vi "ALONE_3AXIS_V_AMI_DESIM_OLD.vi"(6 "Refresco(s)":dbl=1.0, 8 "error in (no error)":errorcluster) -> (0 "Error Out":errorcluster, 7 "Enable":bool=TRUE)   [LabVIEW 2017]
uses:
  AMI MAGNET/Status AMI.ctl
  AMI MAGNET/magneticField.ctl
  ALONE_3AXIS_AMI.ctl
  AMI MAGNET/commsControl.ctl
  AMI MAGNET/AMI 430_Hardware_Module.ctl
  cRIO_ZNB_AMI_GLOBALES.vi
panel:
  out "Ciclo 2":i32
  out "TIEMPO Y":dbl
  out "TIEMPO X":dbl
  out "TIEMPO Z":dbl
  out "cTarget_X":dbl min=-0.5 max=0.5 step=0.001 format="%.3f"
  out "cRate_X":dbl=0.1 min=0.0 max=0.1 step=0.001 format="%.3f"
  out "cTarget_Y":dbl min=-0.5 max=0.5 step=0.001 format="%.3f"
  out "cRate_Y":dbl=0.1 min=0.0 max=0.1 step=0.001 format="%.3f"
  out "ConfigZ":T1={"connection ID"=refnum, "IP"="192.168.0.106", "Active Comm Interface"=0, "Serial Port"="", "Programmer Type"=0, "connection ID"=refnum, "output cluster"={"GPIB address"=22, "GPIB bus"=1}} {"Programmer Type" items=["Model 430", "Model 420"]; "Active Comm Interface" items=["TCP/IP (Model 430 Only)", "RS232", "IEEE488"]}
  out "ConfigY":T1={"connection ID"=refnum, "IP"="192.168.0.107", "Active Comm Interface"=0, "Serial Port"="", "Programmer Type"=0, "connection ID"=refnum, "output cluster"={"GPIB address"=22, "GPIB bus"=1}} {"Programmer Type" items=["Model 430", "Model 420"]; "Active Comm Interface" items=["TCP/IP (Model 430 Only)", "RS232", "IEEE488"]}
  out "ConfigX":T1={"connection ID"=refnum, "IP"="192.168.0.108", "Active Comm Interface"=0, "Serial Port"="", "Programmer Type"=0, "connection ID"=refnum, "output cluster"={"GPIB address"=22, "GPIB bus"=1}} {"Programmer Type" items=["Model 430", "Model 420"]; "Active Comm Interface" items=["TCP/IP (Model 430 Only)", "RS232", "IEEE488"]}
  in  "DEMAG X":bool
  in  "x":dbl=0.1 min=-0.5 max=0.5 step=0.001 format="%.3f"
  in  "y":dbl=0.2 min=-0.5 max=0.5 step=0.001 format="%.3f"
  in  "GO XYZ":bool
  in  "DEMAG Y":bool
  in  "DEMAG Z":bool
  out "Estado":string
  out "Command":T2
  in  "Mode X":u16(ring) items=["RAMP", "PAUSE", "MANUAL UP", "MANUAL DOWN", "ZERO"]
  in  "Mode Y":u16(ring) items=["RAMP", "PAUSE", "MANUAL UP", "MANUAL DOWN", "ZERO"]
  in  "Mode Z":u16(ring) items=["RAMP", "PAUSE", "MANUAL UP", "MANUAL DOWN", "ZERO"]
  in  "GO Z":bool
  in  "SET X":bool
  out "X ramping":bool caption="Stable"
  out "X state":T3=1 items=["Unknown", "RAMPING to target field/current", "HOLDING at the target field/current", "PAUSED", "Ramping in MANUAL UP mode", "Ramping in MANUAL DOWN mode", "ZEROING CURRENT (in progress)", "Quench detected", "At ZERO current", "Heating persistent switch", "Cooling persistent switch", "External Rampdown active"]
  in  "Target X":dbl caption="Target(T)" min=-0.5 max=0.5 step=0.001 format="%.3f"
  in  "Rate X":dbl=0.1 caption="Rate(T/min)" min=0.0 max=0.1 step=0.001 format="%.3f"
  out "X field":dbl caption="X field (T)" format="%.3f"
  in  "SET Y":bool
  out "Y ramping":bool caption="Stable"
  out "Y state":T3=1 items=["Unknown", "RAMPING to target field/current", "HOLDING at the target field/current", "PAUSED", "Ramping in MANUAL UP mode", "Ramping in MANUAL DOWN mode", "ZEROING CURRENT (in progress)", "Quench detected", "At ZERO current", "Heating persistent switch", "Cooling persistent switch", "External Rampdown active"]
  in  "Target Y":dbl caption="Target(T)" min=-0.5 max=0.5 step=0.001 format="%.3f"
  in  "Rate Y":dbl=0.1 caption="Rate(T/min)" min=0.0 max=0.1 step=0.001 format="%.3f"
  out "Y field":dbl caption="Y field (T)" format="%.3f"
  in  "GO X":bool
  in  "GO Y":bool
  in  "Settings Z":T4={"magneticFieldUnits"=1, "rampRateUnits"=1, "rampRate"=0.0, "targetField"=0.0, "rampingMode"=1} {"rampingMode" items=["RAMP", "PAUSE", "MANUAL UP", "MANUAL DOWN", "ZERO"]; "targetField" format="%.3f"; "rampRate" format="%.3f"; "rampRateUnits" items=["Per SECOND", "Per MINUTE"]; "magneticFieldUnits" items=["KGauss", "Tesla"]}
  in  "Settings Y":T4={"magneticFieldUnits"=1, "rampRateUnits"=1, "rampRate"=0.0, "targetField"=0.0, "rampingMode"=1} {"rampingMode" items=["RAMP", "PAUSE", "MANUAL UP", "MANUAL DOWN", "ZERO"]; "targetField" format="%.3f"; "rampRate" format="%.3f"; "rampRateUnits" items=["Per SECOND", "Per MINUTE"]; "magneticFieldUnits" items=["KGauss", "Tesla"]}
  in  "Settings X":T4={"magneticFieldUnits"=1, "rampRateUnits"=1, "rampRate"=0.0, "targetField"=0.0, "rampingMode"=1} {"rampingMode" items=["RAMP", "PAUSE", "MANUAL UP", "MANUAL DOWN", "ZERO"]; "targetField" format="%.3f"; "rampRate" format="%.3f"; "rampRateUnits" items=["Per SECOND", "Per MINUTE"]; "magneticFieldUnits" items=["KGauss", "Tesla"]}
  out "Waveform Chart":T5(graph)
  in  "SET Z":bool
  out "Z ramping":bool caption="Stable"
  out "Z state":T3=1 items=["Unknown", "RAMPING to target field/current", "HOLDING at the target field/current", "PAUSED", "Ramping in MANUAL UP mode", "Ramping in MANUAL DOWN mode", "ZEROING CURRENT (in progress)", "Quench detected", "At ZERO current", "Heating persistent switch", "Cooling persistent switch", "External Rampdown active"]
  out "Ciclo":i32
  in  "Target Z":dbl caption="Target(T)" min=-2.0 max=2.0 step=0.001 format="%.3f"
  in  "Rate Z":dbl=0.1 caption="Rate(T/min)" min=0.0 max=0.1 step=0.001 format="%.3f"
  out "Z field":dbl caption="Z field (T)" format="%.3f"
  out "Error":bool
  out "Date":string
  out "Time":string
  in  "Refresh":bool
  in  "stop":bool
  # "X axis"
  # "Z axis"
  # "STATUS"
  # "Y axis"
  # "STATUS"
  # "STATUS"
  # "SETTINGS"
  # "SETTINGS"
  # "SETTINGS"
  # "-----------X field = x . Z field------------------------------Y field = y . Z field---------------------------- Enlazar con eje Z -------------"
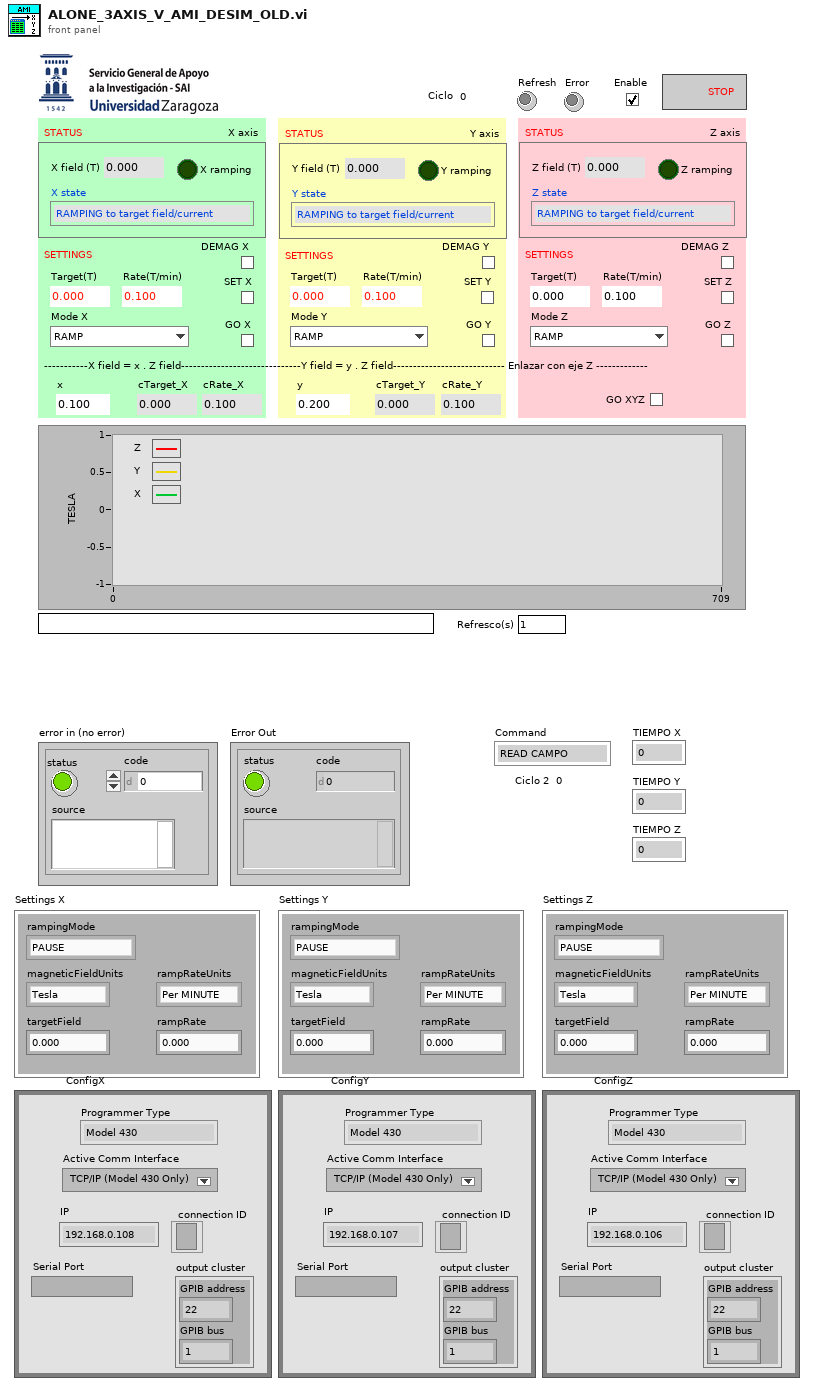
[diagram p1: front panel]
types:
  T1 = typedef "commsControl.ctl" = cluster{"connection ID":refnum<k5>, "IP":string, "Active Comm Interface":u16, "Serial Port":refnum<visa-resource-name>, "Programmer Type":u16, "connection ID":refnum<k5>, "output cluster":cluster{"GPIB address":i16, "GPIB bus":i16}}
  T2 = typedef "ALONE_3AXIS_AMI.ctl" = enum16{"READ CAMPO", "SET X", "SET Y", "SET Z", "RAMP X", "RAMP Y", "RAMP Z", "RAMP XYZ", "DESIMANAR X", "DESIMANAR Y", "DESIMANAR Z", "DESIMANAR X_RUN", "DESIMANAR Y_RUN", "DESIMANAR Z_RUN"}
  T3 = typedef "Status AMI.ctl" = u16
  T4 = typedef "magneticField.ctl" = cluster{"magneticFieldUnits":u16, "rampRateUnits":u16, "rampRate":dbl, "targetField":dbl, "rampingMode":u16}
  T5 = cluster{"magneticField":dbl, "magneticField":dbl, "magneticField":dbl}
  T6 = typedef "AMI 430_Hardware_Module.ctl" = enum16{"INICIALIZAR", "SET UNIDADES CAMPO", "SET UNIDADES RAMPA", "SET CAMPO", "SET  RAMPA", "SET RAMPING MODE", "READ CAMPO", "STATUS", "SHUTDOWN"}
  T7 = cluster{"Z field":dbl, "Y field":dbl, "magneticField":dbl}
  T8 = cluster{"Z field":dbl, "magneticField":dbl, "X field":dbl}
  T9 = cluster{"magneticField":dbl, "Y field":dbl, "X field":dbl}
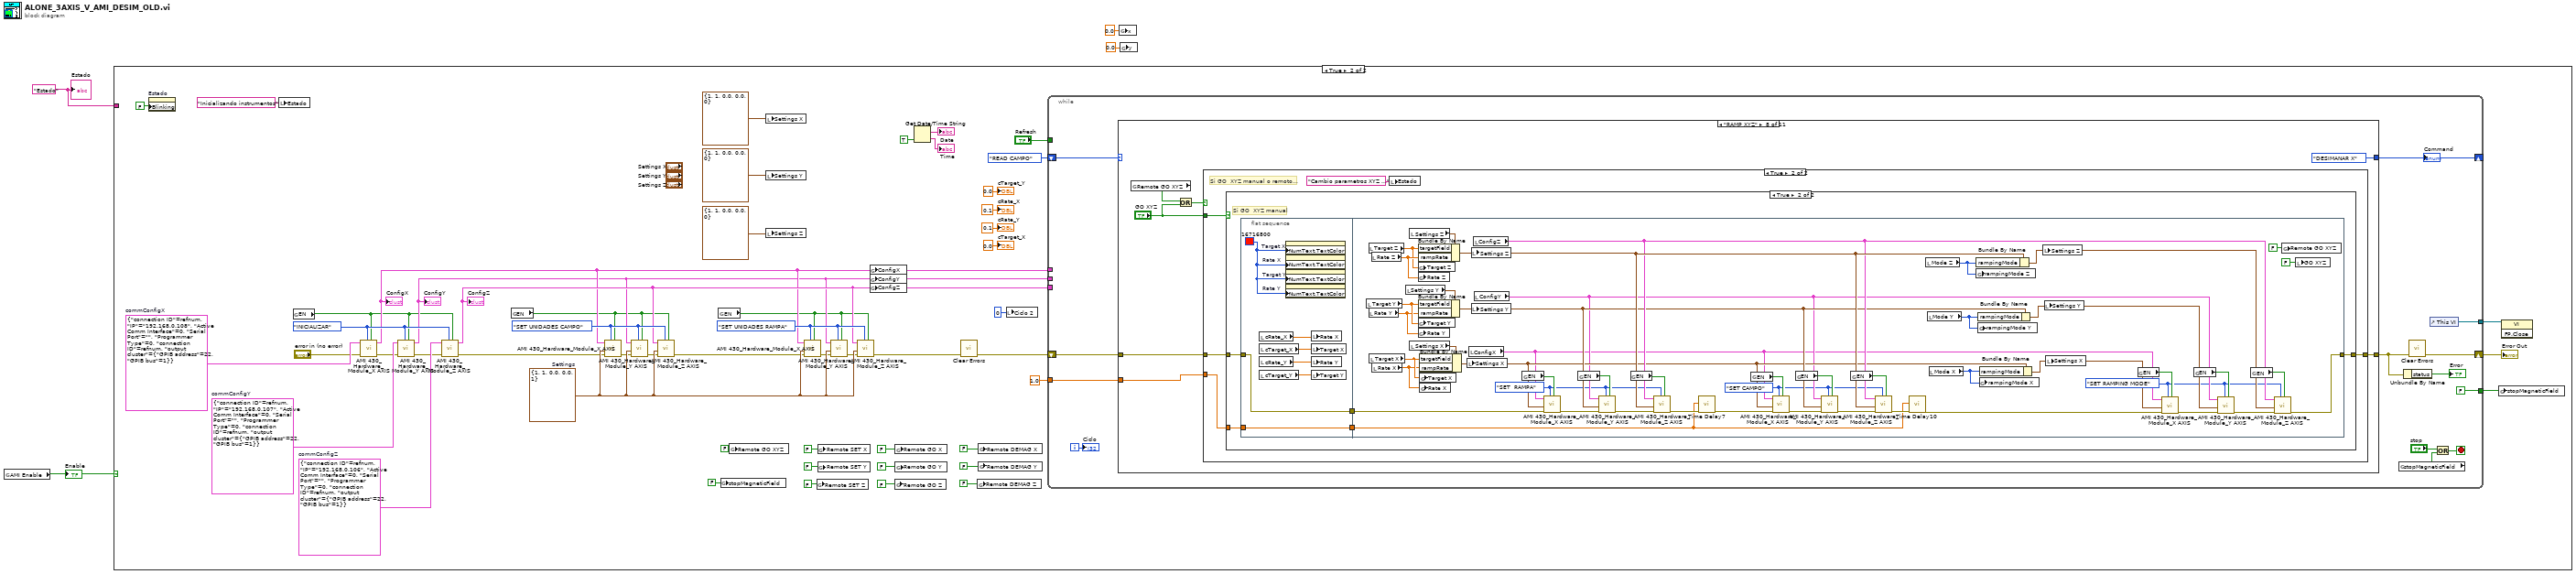
[diagram p0: block diagram]
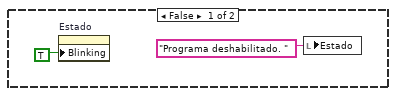
[diagram p2: hidden frame]
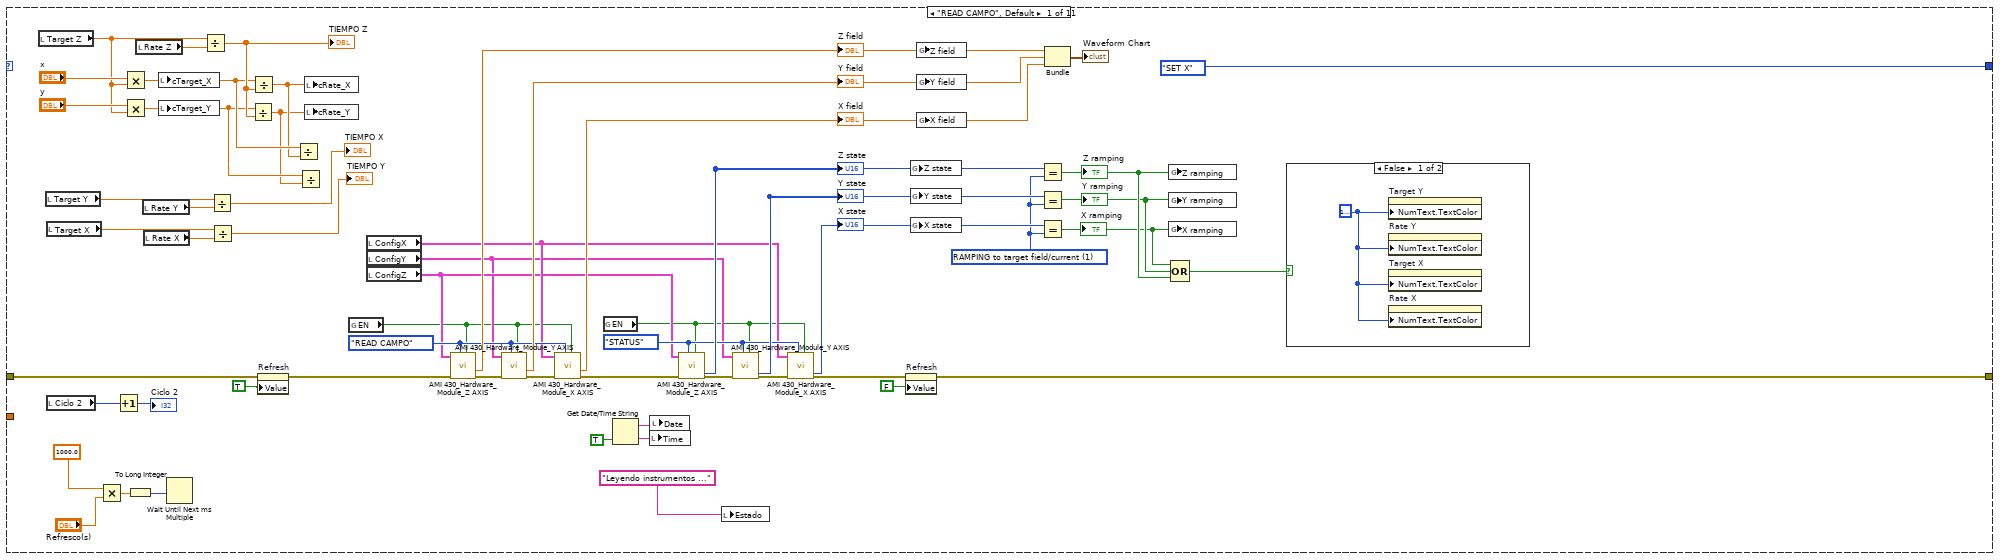
[diagram p3: hidden frame]
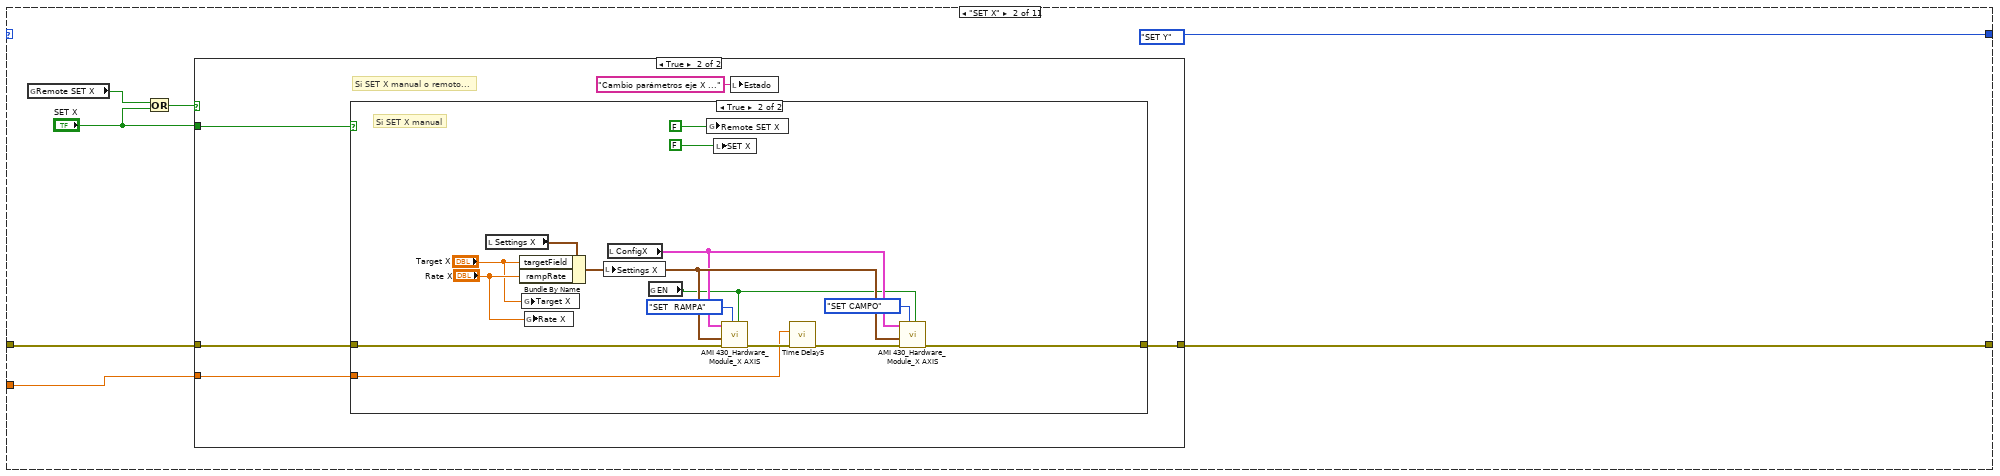
[diagram p5: hidden frame]
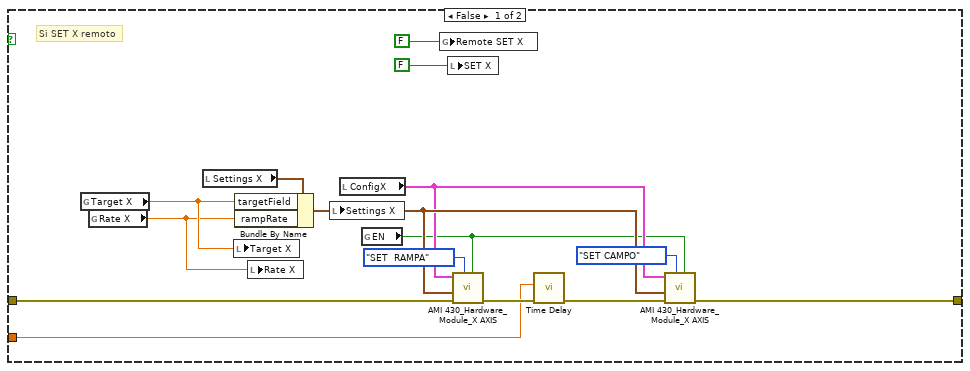
[diagram p7: hidden frame]
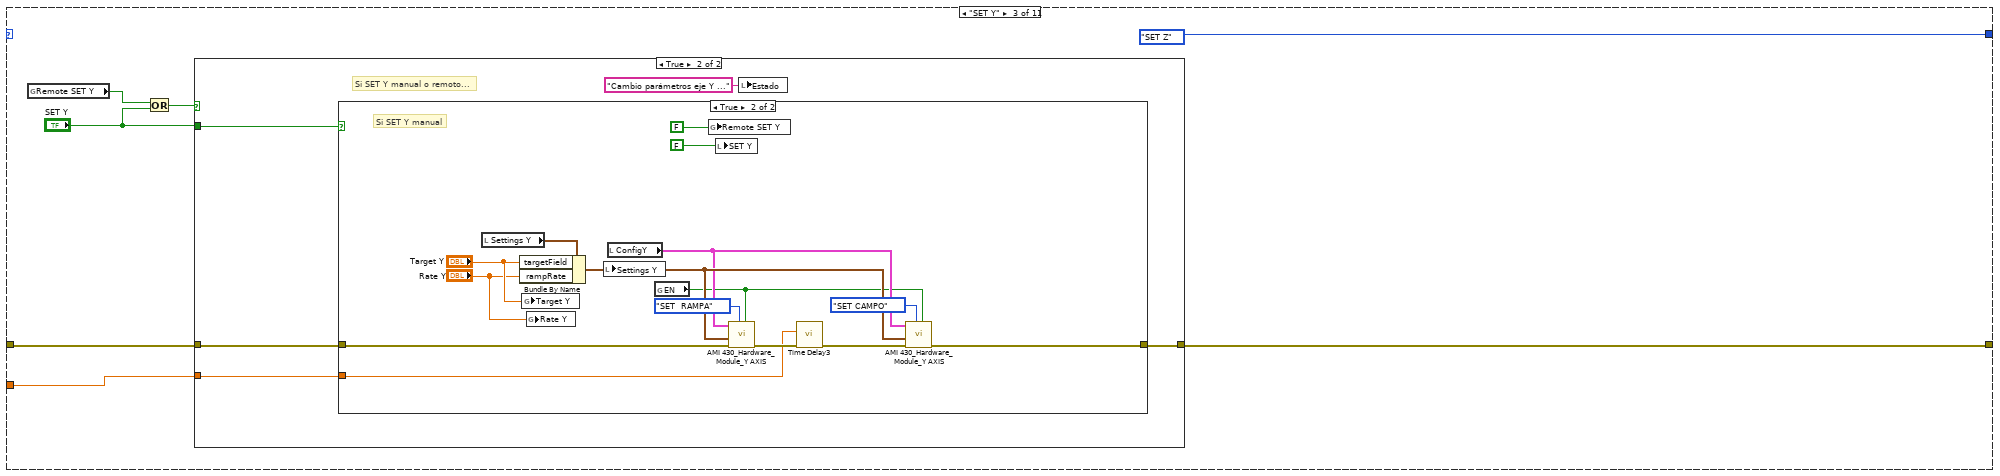
[diagram p8: hidden frame]
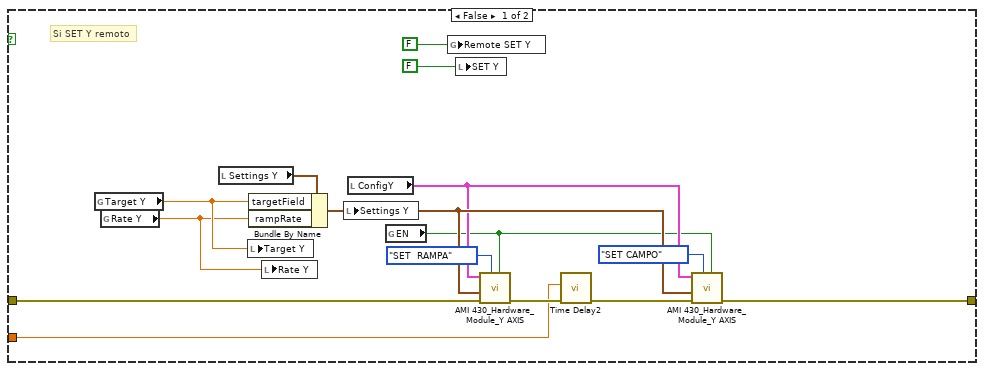
[diagram p10: hidden frame]
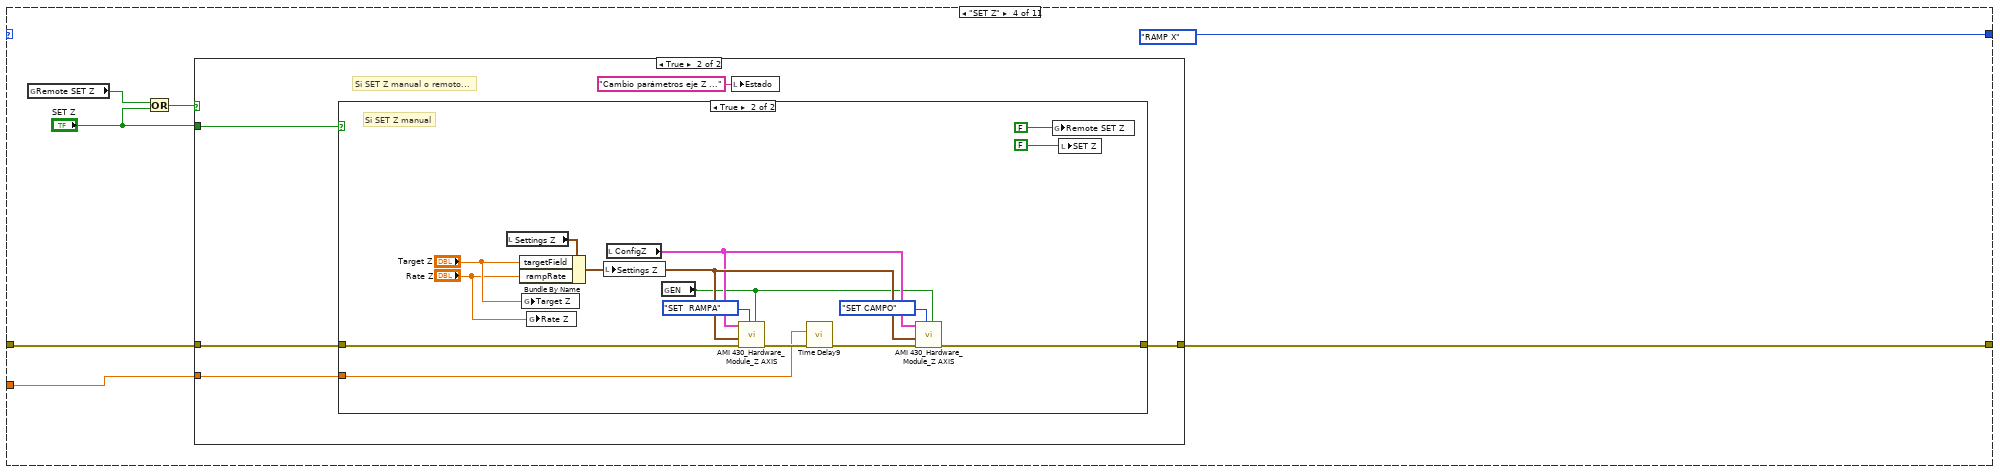
[diagram p11: hidden frame]
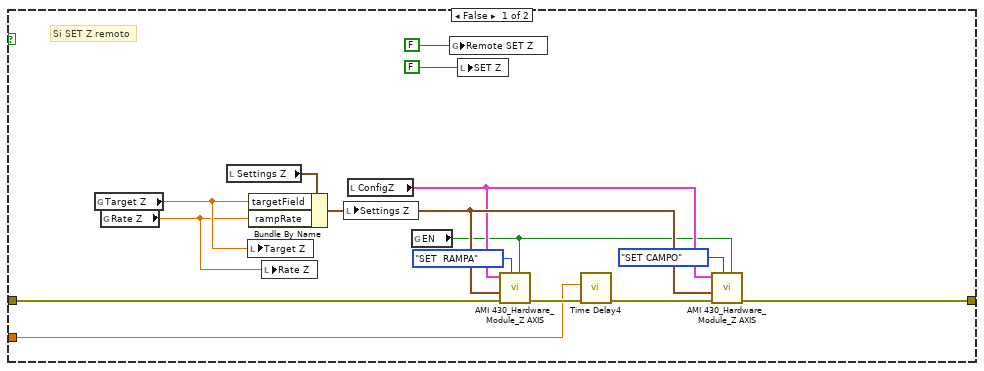
[diagram p13: hidden frame]
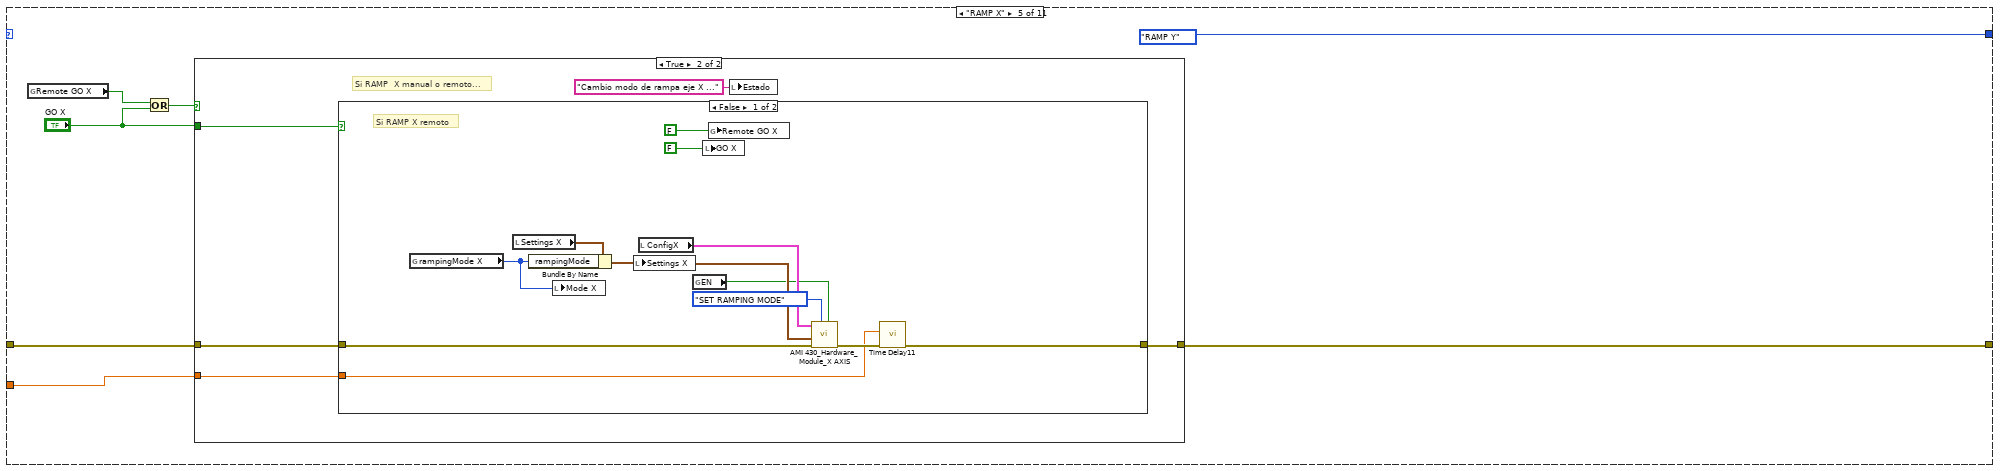
[diagram p14: hidden frame]
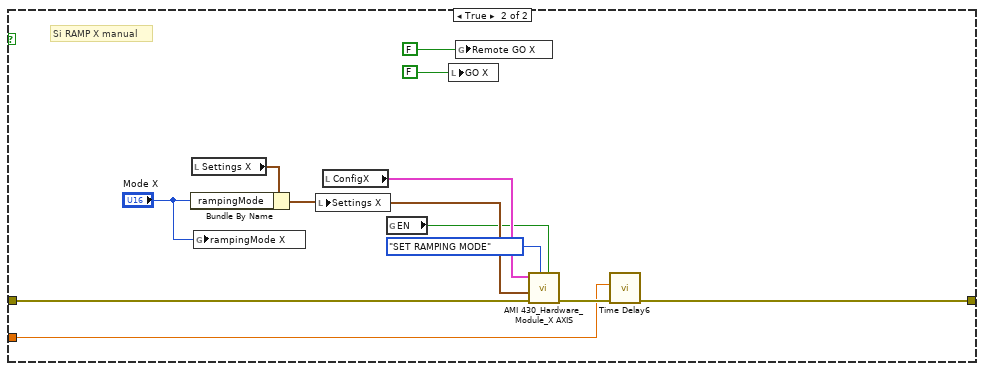
[diagram p16: hidden frame]
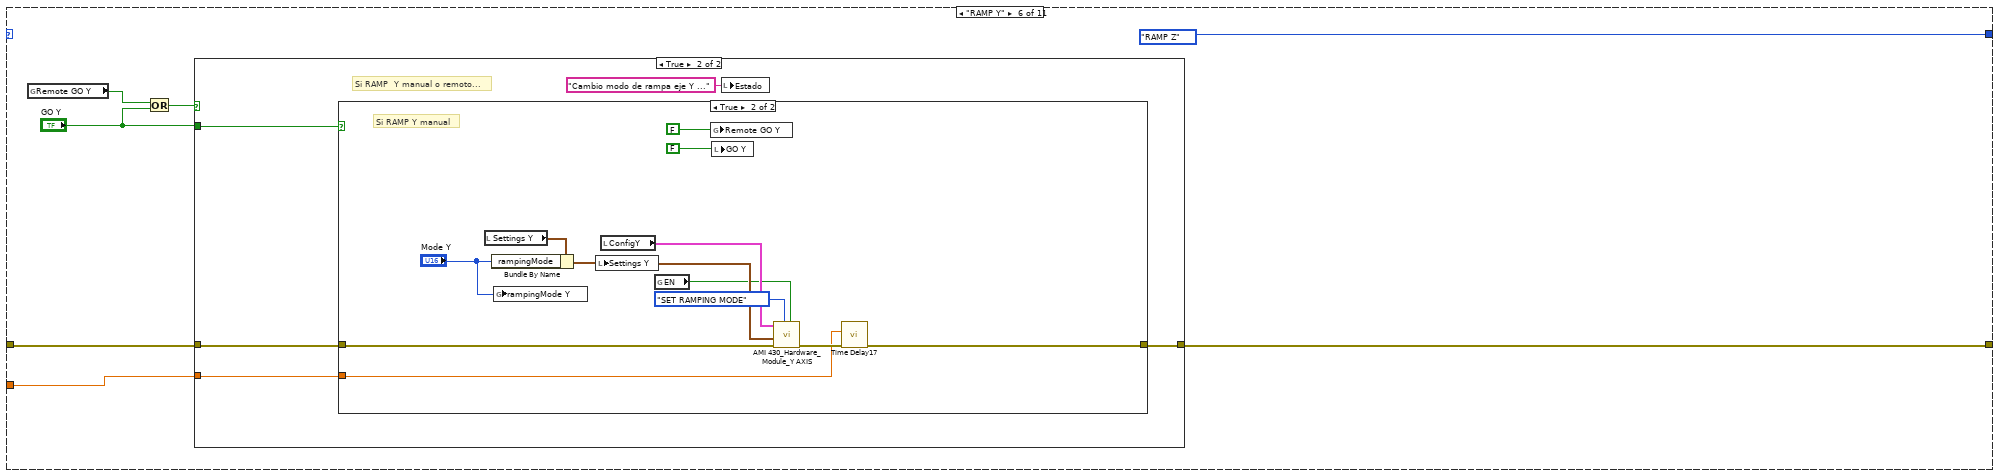
[diagram p17: hidden frame]
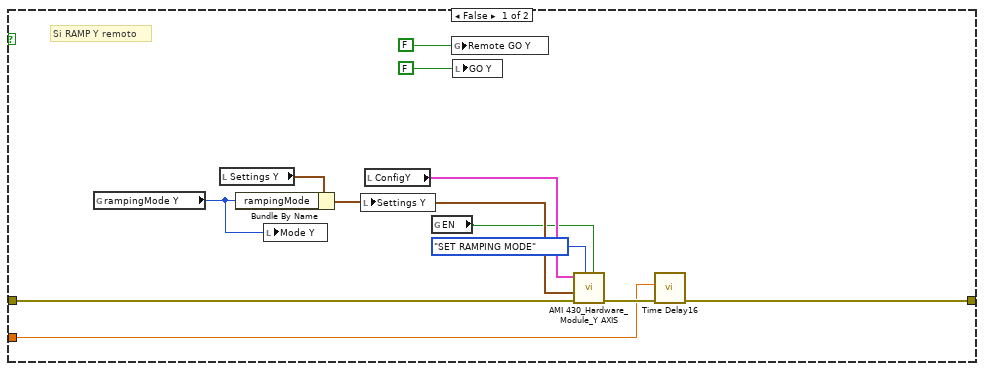
[diagram p19: hidden frame]
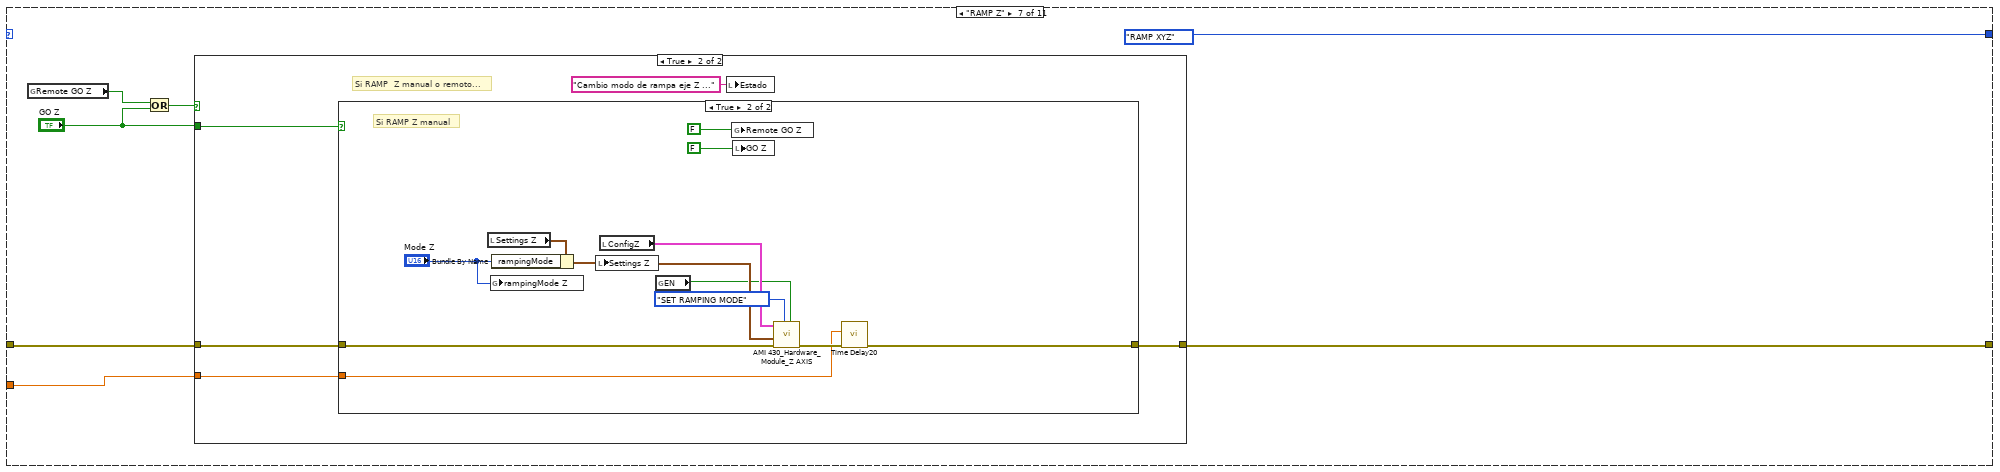
[diagram p20: hidden frame]
diagram:
  w3 = "Estado" ("String")
  n1 = global read "cRIO_ZNB_AMI_GLOBALES.vi" "AMI Enable"() -> (w4:bool)
  "Enable" <- w4
  n2 = case shown="True" w4 {
    tunnel: w3 -> [_ _]
    frame False {
      n3 = property on="Estado" class="Str"("Blinking"=TRUE) -> ()  [unwired: 2 in, 2 out]
      n4 = local write "Estado"("Programa deshabilitado. " ("String")) -> ()
    }
    frame True {
      w53 = T4 {"magneticFieldUnits"=1, "rampRateUnits"=1, "rampRate"=0.0, "targetField"=0.0, "rampingMode"=1}  # Settings
      w49 = AMI_430_Hardware_Module."SET UNIDADES RAMPA" ("Command")
      w48 = AMI_430_Hardware_Module."SET UNIDADES CAMPO" ("Command")
      w56 = T1 {"connection ID"=refnum, "IP"="192.168.0.106", "Active Comm Interface"=0, "Serial Port"="", "Programmer Type"=0, "connection ID"=refnum, "output cluster"={"GPIB address"=22, "GPIB bus"=1}}  # commConfigZ
      w55 = T1 {"connection ID"=refnum, "IP"="192.168.0.107", "Active Comm Interface"=0, "Serial Port"="", "Programmer Type"=0, "connection ID"=refnum, "output cluster"={"GPIB address"=22, "GPIB bus"=1}}  # commConfigY
      w54 = T1 {"connection ID"=refnum, "IP"="192.168.0.108", "Active Comm Interface"=0, "Serial Port"="", "Programmer Type"=0, "connection ID"=refnum, "output cluster"={"GPIB address"=22, "GPIB bus"=1}}  # commConfigX
      w57 = AMI_430_Hardware_Module."INICIALIZAR" ("Command")
      n5 = property on="Estado" class="Str"("Blinking"=FALSE) -> ()  [unwired: 2 in, 2 out]
      n6 = local write "Estado"("Inicializando instrumentos" ("String")) -> ()
      n7 = global read "cRIO_ZNB_AMI_GLOBALES.vi" "EN"() -> (w13:bool)
      n8 = call "AMI 430_Hardware_Module_X AXIS.vi"("Enable"=w13, "Command"=w57, "error in (no error)"="error in (no error)", "Comm Config In"=w54) -> ("error out"=w44:errorcluster, "Comm Config Out"=w22:T1)  [unwired: 3 in, 3 out]
      "ConfigX" <- w22
      n9 = call "AMI 430_Hardware_Module_Y AXIS.vi"("Enable"=w13, "Command"=w57, "error in (no error)"=w44, "Comm Config In"=w55) -> ("error out"=w43:errorcluster, "Comm Config Out"=w21:T1)  [unwired: 3 in, 3 out]
      "ConfigY" <- w21
      n10 = call "AMI 430_Hardware_Module_Z AXIS.vi"("Enable"=w13, "Command"=w57, "error in (no error)"=w43, "Comm Config In"=w56) -> ("error out"=w47:errorcluster, "Comm Config Out"=w23:T1)  [unwired: 3 in, 3 out]
      "ConfigZ" <- w23
      n11 = global read "cRIO_ZNB_AMI_GLOBALES.vi" "EN"() -> (w12:bool)
      n12 = call "AMI 430_Hardware_Module_X AXIS.vi"("Enable"=w12, "Command"=w48, "error in (no error)"=w47, "Settings"=w53, "Comm Config In"=w22) -> ("error out"=w45:errorcluster)  [unwired: 2 in, 4 out]
      n13 = call "AMI 430_Hardware_Module_Y AXIS.vi"("Enable"=w12, "Command"=w48, "error in (no error)"=w45, "Settings"=w53, "Comm Config In"=w21) -> ("error out"=w46:errorcluster)  [unwired: 2 in, 4 out]
      n14 = call "AMI 430_Hardware_Module_Z AXIS.vi"("Enable"=w12, "Command"=w48, "error in (no error)"=w46, "Settings"=w53, "Comm Config In"=w23) -> ("error out"=w52:errorcluster)  [unwired: 2 in, 4 out]
      n15 = global read "cRIO_ZNB_AMI_GLOBALES.vi" "EN"() -> (w11:bool)
      n16 = global write "cRIO_ZNB_AMI_GLOBALES.vi" "stopMagneticField"(FALSE ("stopMagneticField")) -> ()
      n17 = global write "cRIO_ZNB_AMI_GLOBALES.vi" "Remote GO XYZ"(FALSE ("Remote SET Z")) -> ()
      n18 = local write "Settings X"(T4 {"magneticFieldUnits"=1, "rampRateUnits"=1, "rampRate"=0.0, "targetField"=0.0, "rampingMode"=0} ("Settings X")) -> ()
      n19 = local write "Settings Y"(T4 {"magneticFieldUnits"=1, "rampRateUnits"=1, "rampRate"=0.0, "targetField"=0.0, "rampingMode"=0} ("Settings Y")) -> ()
      n20 = local write "Settings Z"(T4 {"magneticFieldUnits"=1, "rampRateUnits"=1, "rampRate"=0.0, "targetField"=0.0, "rampingMode"=0} ("Settings Z")) -> ()
      n21 = call "AMI 430_Hardware_Module_X AXIS.vi"("Enable"=w11, "Command"=w49, "error in (no error)"=w52, "Settings"=w53, "Comm Config In"=w22) -> ("error out"=w50:errorcluster)  [unwired: 2 in, 4 out]
      n22 = global write "cRIO_ZNB_AMI_GLOBALES.vi" "Remote SET Z"(FALSE ("Remote SET Z")) -> ()
      n23 = global write "cRIO_ZNB_AMI_GLOBALES.vi" "Remote SET X"(FALSE ("Remote SET X")) -> ()
      n24 = global write "cRIO_ZNB_AMI_GLOBALES.vi" "Remote SET Y"(FALSE ("Remote SET Y")) -> ()
      n25 = call "AMI 430_Hardware_Module_Y AXIS.vi"("Enable"=w11, "Command"=w49, "error in (no error)"=w50, "Settings"=w53, "Comm Config In"=w21) -> ("error out"=w51:errorcluster)  [unwired: 2 in, 4 out]
      n26 = call "AMI 430_Hardware_Module_Z AXIS.vi"("Enable"=w11, "Command"=w49, "error in (no error)"=w51, "Settings"=w53, "Comm Config In"=w23) -> ("error out"=w42:errorcluster)  [unwired: 2 in, 4 out]
      n27 = global write "cRIO_ZNB_AMI_GLOBALES.vi" "ConfigX"(w22) -> ()
      n28 = global write "cRIO_ZNB_AMI_GLOBALES.vi" "ConfigY"(w21) -> ()
      n29 = global write "cRIO_ZNB_AMI_GLOBALES.vi" "ConfigZ"(w23) -> ()
      n30 = global write "cRIO_ZNB_AMI_GLOBALES.vi" "Remote GO Z"(FALSE ("Remote RAMP Z")) -> ()
      n31 = global write "cRIO_ZNB_AMI_GLOBALES.vi" "Remote GO X"(FALSE ("Remote RAMP X")) -> ()
      n32 = global write "cRIO_ZNB_AMI_GLOBALES.vi" "Remote GO Y"(FALSE ("Remote RAMP Y")) -> ()
      n33 = Get Date/Time String(want seconds? (F)=TRUE) -> (date string=→"Date":string, time string=→"Time":string)  [unwired: 2 in]
      n34 = call <vilib>:"Clear Errors.vi"("error in (no error)"=w42) -> ("error out"=w38:errorcluster)  [unwired: 5 in, 1 out]
      n35 = global write "cRIO_ZNB_AMI_GLOBALES.vi" "Remote DEMAG Z"(FALSE ("Remote RAMP Z")) -> ()
      n36 = global write "cRIO_ZNB_AMI_GLOBALES.vi" "Remote DEMAG X"(FALSE ("Remote RAMP X")) -> ()
      n37 = global write "cRIO_ZNB_AMI_GLOBALES.vi" "Remote DEMAG Y"(FALSE ("Remote RAMP Y")) -> ()
      n38 = local write "Ciclo 2"(0 ("Ciclo 2")) -> ()
      n39 = while {
        shift-right: [w67] -> w58
        shift-left: w38 -> [w63]
        tunnel: [FALSE ("stop")] -> w59
        tunnel: [w70] -> w60
        tunnel: "Refresh" -> [_]
        tunnel: w21 -> [_]
        tunnel: w23 -> [_]
        tunnel: w22 -> [_]
        shift-right: [w62] -> _
        shift-left: ALONE_3AXIS_AMI."READ CAMPO" ("Command") -> [w65]
        tunnel: 1.0 ("Delay Time (s)") -> [w61]
        i -> [w66]
        stop <- w72 stop-if-true
        n40 = case shown="\"RAMP XYZ\"" w65 {
          tunnel: w63 -> [w106 w137 w180 w223 w266 w303 w340 w377 w451 w525 w599]
          tunnel: [w103 w136 w179 w222 w265 w302 w339 w376 w450 w524 w598] -> w64
          tunnel: [ALONE_3AXIS_AMI."SET X" ("Command") ALONE_3AXIS_AMI."SET Y" ("Command") ALONE_3AXIS_AMI."SET Z" ("Command") ALONE_3AXIS_AMI."RAMP X" ("Command") ALONE_3AXIS_AMI."RAMP Y" ("Command") ALONE_3AXIS_AMI."RAMP Z" ("Command") ALONE_3AXIS_AMI."RAMP XYZ" ("Command") ALONE_3AXIS_AMI."DESIMANAR X" ("Command") ALONE_3AXIS_AMI."DESIMANAR Y" ("Command") ALONE_3AXIS_AMI."DESIMANAR Z" ("Command") ALONE_3AXIS_AMI."READ CAMPO" ("Command")] -> w62
          tunnel: w61 -> [_ w134 w177 w220 w263 w300 w338 w375 w448 w522 w596]
          frame "READ CAMPO", Default {
            w117 = T3 1 items=["Unknown", "RAMPING to target field/current", "HOLDING at the target field/current", "PAUSED", "Ramping in MANUAL UP mode", "Ramping in MANUAL DOWN mode", "ZEROING CURRENT (in progress)", "Quench detected", "At ZERO current", "Heating persistent switch", "Cooling persistent switch", "External Rampdown active"] ("y")
            w116 = AMI_430_Hardware_Module."STATUS" ("Command")
            w115 = AMI_430_Hardware_Module."READ CAMPO" ("Command")
            n41 = local read "Target Z"() -> (w92:dbl)
            n42 = local read "Target Y"() -> (w78:dbl)
            n43 = local read "Target X"() -> (w77:dbl)
            n44 = local read "Ciclo 2"() -> (w85:i32)
            n45 = Multiply(x=1000.0, y="Refresco(s)") -> (x*y=w111:dbl)
            n46 = Increment(x=w85) -> (x+1=→"Ciclo 2":i32)
            n47 = Multiply(x="x", y=w92) -> (x*y=w89:dbl)
            n48 = Multiply(x="y", y=w92) -> (x*y=w88:dbl)
            n49 = To Long Integer(number=w111) -> (32bit integer=w109:i32)
            n50 = local read "Rate Z"() -> (w91:dbl)
            n51 = local read "Rate Y"() -> (w79:dbl)
            n52 = local read "Rate X"() -> (w76:dbl)
            n53 = local write "cTarget_X"(w89) -> ()
            n54 = local write "cTarget_Y"(w88) -> ()
            n55 = Wait Until Next ms Multiple(millisecond multiple=w109) -> ()  [unwired: 1 out]
            n56 = Divide(x=w92, y=w91) -> (x/y=w90:dbl)
            "TIEMPO Z" <- w90
            n57 = Divide(x=w78, y=w79) -> (x/y=→"TIEMPO X":dbl)
            n58 = Divide(x=w77, y=w76) -> (x/y=→"TIEMPO Y":dbl)
            n59 = Divide(x=w88, y=w90) -> (x/y=w86:dbl)
            n60 = Divide(x=w89, y=w90) -> (x/y=w87:dbl)
            n61 = property on="Refresh" class="Bool (strict)"(error in=w106, "Value"=TRUE ("Refresh")) -> (error out=w105:errorcluster)  [unwired: 1 in, 1 out]
            n62 = Divide(x=w89, y=w87) -> ()  [unwired: 1 out]
            n63 = Divide(x=w88, y=w86) -> ()  [unwired: 1 out]
            n64 = local write "cRate_X"(w87) -> ()
            n65 = local write "cRate_Y"(w86) -> ()
            n66 = global read "cRIO_ZNB_AMI_GLOBALES.vi" "EN"() -> (w96:bool)
            n67 = local read "ConfigX"() -> (w102:T1)
            n68 = local read "ConfigY"() -> (w100:T1)
            n69 = local read "ConfigZ"() -> (w101:T1)
            n70 = call "AMI 430_Hardware_Module_Z AXIS.vi"("Enable"=w96, "Command"=w115, "error in (no error)"=w105, "Comm Config In"=w101) -> ("error out"=w119:errorcluster, "magneticField"=w126:dbl)  [unwired: 3 in, 3 out]
            "Z field" <- w126
            n71 = call "AMI 430_Hardware_Module_Y AXIS.vi"("Enable"=w96, "Command"=w115, "error in (no error)"=w119, "Comm Config In"=w100) -> ("error out"=w118:errorcluster, "magneticField"=w125:dbl)  [unwired: 3 in, 3 out]
            "Y field" <- w125
            n72 = call "AMI 430_Hardware_Module_X AXIS.vi"("Enable"=w96, "Command"=w115, "error in (no error)"=w118, "Comm Config In"=w102) -> ("error out"=w120:errorcluster, "magneticField"=w124:dbl)  [unwired: 3 in, 3 out]
            "X field" <- w124
            n73 = global read "cRIO_ZNB_AMI_GLOBALES.vi" "EN"() -> (w95:bool)
            n74 = Get Date/Time String(want seconds? (F)=TRUE) -> (date string=w98:string, time string=w97:string)  [unwired: 2 in]
            n75 = local write "Time"(w97) -> ()
            n76 = local write "Date"(w98) -> ()
            n77 = call "AMI 430_Hardware_Module_Z AXIS.vi"("Enable"=w95, "Command"=w116, "error in (no error)"=w120, "Comm Config In"=w101) -> ("error out"=w122:errorcluster, "state"=w127:T3)  [unwired: 3 in, 3 out]
            "Z state" <- w127
            n78 = local write "Estado"("Leyendo instrumentos ..." ("String")) -> ()
            n79 = call "AMI 430_Hardware_Module_Y AXIS.vi"("Enable"=w95, "Command"=w116, "error in (no error)"=w122, "Comm Config In"=w100) -> ("error out"=w121:errorcluster, "state"=w128:T3)  [unwired: 3 in, 3 out]
            "Y state" <- w128
            n80 = call "AMI 430_Hardware_Module_X AXIS.vi"("Enable"=w95, "Command"=w116, "error in (no error)"=w121, "Comm Config In"=w102) -> ("error out"=w104:errorcluster, "state"=w129:T3)  [unwired: 3 in, 3 out]
            "X state" <- w129
            n81 = property on="Refresh" class="Bool (strict)"(error in=w104, "Value"=FALSE ("Refresh")) -> (error out=w103:errorcluster)  [unwired: 1 in, 1 out]
            n82 = global write "cRIO_ZNB_AMI_GLOBALES.vi" "Z state"(w127) -> ()
            n83 = global write "cRIO_ZNB_AMI_GLOBALES.vi" "Y state"(w128) -> ()
            n84 = global write "cRIO_ZNB_AMI_GLOBALES.vi" "X state"(w129) -> ()
            n85 = global write "cRIO_ZNB_AMI_GLOBALES.vi" "Z field"(w126) -> ()
            n86 = global write "cRIO_ZNB_AMI_GLOBALES.vi" "Y field"(w125) -> ()
            n87 = global write "cRIO_ZNB_AMI_GLOBALES.vi" "X field"(w124) -> ()
            n88 = Equal?(x=w127, y=w117) -> (x = y?=w83:bool)
            "Z ramping" <- w83
            n89 = Equal?(x=w128, y=w117) -> (x = y?=w82:bool)
            "Y ramping" <- w82
            n90 = Equal?(x=w129, y=w117) -> (x = y?=w81:bool)
            "X ramping" <- w81
            n91 = Bundle("magneticField"=w126, "magneticField"=w125, "magneticField"=w124) -> (→"Waveform Chart":T5)  [unwired: 1 in]
            n92 = global write "cRIO_ZNB_AMI_GLOBALES.vi" "Z ramping"(w83) -> ()
            n93 = global write "cRIO_ZNB_AMI_GLOBALES.vi" "Y ramping"(w82) -> ()
            n94 = global write "cRIO_ZNB_AMI_GLOBALES.vi" "X ramping"(w81) -> ()
            n95 = Compound Arithmetic op=OR(w81, w82, w83) -> (w80:bool)
            n96 = case shown="False" w80 {
              frame False {
                w130 = u32 16777222 ("Color Box 2")
                n97 = property on="Target Y" class="DigNum (strict)"("NumText.TextColor"=w130) -> ()  [unwired: 2 in, 2 out]
                n98 = property on="Rate Y" class="DigNum (strict)"("NumText.TextColor"=w130) -> ()  [unwired: 2 in, 2 out]
                n99 = property on="Target X" class="DigNum (strict)"("NumText.TextColor"=w130) -> ()  [unwired: 2 in, 2 out]
                n100 = property on="Rate X" class="DigNum (strict)"("NumText.TextColor"=w130) -> ()  [unwired: 2 in, 2 out]
              }
              frame True {
              }
            }
          }
          frame "SET X" {
            n101 = global read "cRIO_ZNB_AMI_GLOBALES.vi" "Remote SET X"() -> (w133:bool)
            n102 = Or(x=w133, y="SET X") -> (x .or. y?=w132:bool)
            n103 = case shown="True" w132 {
              tunnel: w137 -> [w138 w143]
              tunnel: [w138 w142] -> w136
              tunnel: w134 -> [_ w141]
              tunnel: "SET X" -> [_ w140]
              frame False {
              }
              frame True {
                # "Si SET X manual o remoto..."
                n104 = case shown="True" w140 {
                  tunnel: w143 -> [w153 w166]
                  tunnel: [w152 w165] -> w142
                  tunnel: w141 -> [w151 w164]
                  frame False {
                    # "Si SET X remoto"
                    n105 = global read "cRIO_ZNB_AMI_GLOBALES.vi" "Target X"() -> (w150:dbl)
                    n106 = global read "cRIO_ZNB_AMI_GLOBALES.vi" "Rate X"() -> (w149:dbl)
                    n107 = local read "Settings X"() -> (w144:T4)
                    n108 = local write "Target X"(w150) -> ()
                    n109 = Bundle By Name(cluster=w144, "targetField"=w150, "rampRate"=w149) -> (w158:T4)
                    n110 = local write "Rate X"(w149) -> ()
                    n111 = local write "Settings X"(w158) -> ()
                    n112 = local read "ConfigX"() -> (w146:T1)
                    n113 = global read "cRIO_ZNB_AMI_GLOBALES.vi" "EN"() -> (w145:bool)
                    n114 = global write "cRIO_ZNB_AMI_GLOBALES.vi" "Remote SET X"(FALSE ("Remote SET X")) -> ()
                    n115 = local write "SET X"(FALSE ("Remote SET X")) -> ()
                    n116 = call "AMI 430_Hardware_Module_X AXIS.vi"("Enable"=w145, "Command"=AMI_430_Hardware_Module."SET  RAMPA", "error in (no error)"=w153, "Settings"=w158, "Comm Config In"=w146) -> ("error out"=w156:errorcluster)  [unwired: 2 in, 4 out]
                    n117 = call "Time Delay"("error in (no error)"=w156, "Delay Time (s)"=w151) -> ("error out"=w157:errorcluster)  [unwired: 9 in]
                    n118 = call "AMI 430_Hardware_Module_X AXIS.vi"("Enable"=w145, "Command"=AMI_430_Hardware_Module."SET CAMPO", "error in (no error)"=w157, "Settings"=w158, "Comm Config In"=w146) -> ("error out"=w152:errorcluster)  [unwired: 2 in, 4 out]
                  }
                  frame True {
                    # "Si SET X manual"
                    n119 = local read "Settings X"() -> (w159:T4)
                    n120 = Bundle By Name(cluster=w159, "targetField"="Target X", "rampRate"="Rate X") -> (w171:T4)
                    n121 = global write "cRIO_ZNB_AMI_GLOBALES.vi" "Target X"("Target X") -> ()
                    n122 = global write "cRIO_ZNB_AMI_GLOBALES.vi" "Rate X"("Rate X") -> ()
                    n123 = local write "Settings X"(w171) -> ()
                    n124 = local read "ConfigX"() -> (w161:T1)
                    n125 = global read "cRIO_ZNB_AMI_GLOBALES.vi" "EN"() -> (w160:bool)
                    n126 = global write "cRIO_ZNB_AMI_GLOBALES.vi" "Remote SET X"(FALSE ("Remote SET X")) -> ()
                    n127 = local write "SET X"(FALSE ("Remote SET X")) -> ()
                    n128 = call "AMI 430_Hardware_Module_X AXIS.vi"("Enable"=w160, "Command"=AMI_430_Hardware_Module."SET  RAMPA", "error in (no error)"=w166, "Settings"=w171, "Comm Config In"=w161) -> ("error out"=w169:errorcluster)  [unwired: 2 in, 4 out]
                    n129 = call "Time Delay5"("error in (no error)"=w169, "Delay Time (s)"=w164) -> ("error out"=w170:errorcluster)  [unwired: 9 in]
                    n130 = call "AMI 430_Hardware_Module_X AXIS.vi"("Enable"=w160, "Command"=AMI_430_Hardware_Module."SET CAMPO", "error in (no error)"=w170, "Settings"=w171, "Comm Config In"=w161) -> ("error out"=w165:errorcluster)  [unwired: 2 in, 4 out]
                  }
                }
                n131 = local write "Estado"("Cambio parámetros eje X ..." ("String")) -> ()
              }
            }
          }
          frame "SET Y" {
            n132 = global read "cRIO_ZNB_AMI_GLOBALES.vi" "Remote SET Y"() -> (w176:bool)
            n133 = Or(x=w176, y="SET Y") -> (x .or. y?=w175:bool)
            n134 = case shown="True" w175 {
              tunnel: w180 -> [w181 w186]
              tunnel: [w181 w185] -> w179
              tunnel: w177 -> [_ w184]
              tunnel: "SET Y" -> [_ w183]
              frame False {
              }
              frame True {
                # "Si SET Y manual o remoto..."
                n135 = case shown="True" w183 {
                  tunnel: w186 -> [w192 w210]
                  tunnel: [w190 w209] -> w185
                  tunnel: w184 -> [w191 w208]
                  frame False {
                    # "Si SET Y remoto"
                    n136 = global read "cRIO_ZNB_AMI_GLOBALES.vi" "Target Y"() -> (w201:dbl)
                    n137 = global read "cRIO_ZNB_AMI_GLOBALES.vi" "Rate Y"() -> (w200:dbl)
                    n138 = local read "Settings Y"() -> (w187:T4)
                    n139 = local write "Target Y"(w201) -> ()
                    n140 = Bundle By Name(cluster=w187, "targetField"=w201, "rampRate"=w200) -> (w193:T4)
                    n141 = local write "Rate Y"(w200) -> ()
                    n142 = local write "Settings Y"(w193) -> ()
                    n143 = local read "ConfigY"() -> (w189:T1)
                    n144 = global read "cRIO_ZNB_AMI_GLOBALES.vi" "EN"() -> (w188:bool)
                    n145 = global write "cRIO_ZNB_AMI_GLOBALES.vi" "Remote SET Y"(FALSE ("Remote SET X")) -> ()
                    n146 = local write "SET Y"(FALSE ("Remote SET X")) -> ()
                    n147 = call "AMI 430_Hardware_Module_Y AXIS.vi"("Enable"=w188, "Command"=AMI_430_Hardware_Module."SET  RAMPA", "error in (no error)"=w192, "Settings"=w193, "Comm Config In"=w189) -> ("error out"=w197:errorcluster)  [unwired: 2 in, 4 out]
                    n148 = call "Time Delay2"("error in (no error)"=w197, "Delay Time (s)"=w191) -> ("error out"=w195:errorcluster)  [unwired: 9 in]
                    n149 = call "AMI 430_Hardware_Module_Y AXIS.vi"("Enable"=w188, "Command"=AMI_430_Hardware_Module."SET CAMPO", "error in (no error)"=w195, "Settings"=w193, "Comm Config In"=w189) -> ("error out"=w190:errorcluster)  [unwired: 2 in, 4 out]
                  }
                  frame True {
                    # "Si SET Y manual"
                    n150 = local read "Settings Y"() -> (w202:T4)
                    n151 = Bundle By Name(cluster=w202, "targetField"="Target Y", "rampRate"="Rate Y") -> (w207:T4)
                    n152 = global write "cRIO_ZNB_AMI_GLOBALES.vi" "Target Y"("Target Y") -> ()
                    n153 = global write "cRIO_ZNB_AMI_GLOBALES.vi" "Rate Y"("Rate Y") -> ()
                    n154 = local write "Settings Y"(w207) -> ()
                    n155 = local read "ConfigY"() -> (w204:T1)
                    n156 = global read "cRIO_ZNB_AMI_GLOBALES.vi" "EN"() -> (w203:bool)
                    n157 = global write "cRIO_ZNB_AMI_GLOBALES.vi" "Remote SET Y"(FALSE ("Remote SET X")) -> ()
                    n158 = local write "SET Y"(FALSE ("Remote SET X")) -> ()
                    n159 = call "AMI 430_Hardware_Module_Y AXIS.vi"("Enable"=w203, "Command"=AMI_430_Hardware_Module."SET  RAMPA", "error in (no error)"=w210, "Settings"=w207, "Comm Config In"=w204) -> ("error out"=w214:errorcluster)  [unwired: 2 in, 4 out]
                    n160 = call "Time Delay3"("error in (no error)"=w214, "Delay Time (s)"=w208) -> ("error out"=w212:errorcluster)  [unwired: 9 in]
                    n161 = call "AMI 430_Hardware_Module_Y AXIS.vi"("Enable"=w203, "Command"=AMI_430_Hardware_Module."SET CAMPO", "error in (no error)"=w212, "Settings"=w207, "Comm Config In"=w204) -> ("error out"=w209:errorcluster)  [unwired: 2 in, 4 out]
                  }
                }
                n162 = local write "Estado"("Cambio parámetros eje Y ..." ("String")) -> ()
              }
            }
          }
          frame "SET Z" {
            n163 = global read "cRIO_ZNB_AMI_GLOBALES.vi" "Remote SET Z"() -> (w219:bool)
            n164 = Or(x=w219, y="SET Z") -> (x .or. y?=w218:bool)
            n165 = case shown="True" w218 {
              tunnel: w223 -> [w224 w229]
              tunnel: [w224 w228] -> w222
              tunnel: w220 -> [_ w227]
              tunnel: "SET Z" -> [_ w226]
              frame False {
              }
              frame True {
                # "Si SET Z manual o remoto..."
                n166 = case shown="True" w226 {
                  tunnel: w229 -> [w235 w253]
                  tunnel: [w234 w252] -> w228
                  tunnel: w227 -> [w236 w250]
                  frame False {
                    # "Si SET Z remoto"
                    n167 = global read "cRIO_ZNB_AMI_GLOBALES.vi" "Target Z"() -> (w244:dbl)
                    n168 = global read "cRIO_ZNB_AMI_GLOBALES.vi" "Rate Z"() -> (w243:dbl)
                    n169 = local read "Settings Z"() -> (w230:T4)
                    n170 = local write "Target Z"(w244) -> ()
                    n171 = Bundle By Name(cluster=w230, "targetField"=w244, "rampRate"=w243) -> (w233:T4)
                    n172 = local write "Rate Z"(w243) -> ()
                    n173 = local write "Settings Z"(w233) -> ()
                    n174 = local read "ConfigZ"() -> (w232:T1)
                    n175 = global read "cRIO_ZNB_AMI_GLOBALES.vi" "EN"() -> (w231:bool)
                    n176 = global write "cRIO_ZNB_AMI_GLOBALES.vi" "Remote SET Z"(FALSE ("Remote SET X")) -> ()
                    n177 = local write "SET Z"(FALSE ("Remote SET X")) -> ()
                    n178 = call "AMI 430_Hardware_Module_Z AXIS.vi"("Enable"=w231, "Command"=AMI_430_Hardware_Module."SET  RAMPA", "error in (no error)"=w235, "Settings"=w233, "Comm Config In"=w232) -> ("error out"=w238:errorcluster)  [unwired: 2 in, 4 out]
                    n179 = call "Time Delay4"("error in (no error)"=w238, "Delay Time (s)"=w236) -> ("error out"=w237:errorcluster)  [unwired: 9 in]
                    n180 = call "AMI 430_Hardware_Module_Z AXIS.vi"("Enable"=w231, "Command"=AMI_430_Hardware_Module."SET CAMPO", "error in (no error)"=w237, "Settings"=w233, "Comm Config In"=w232) -> ("error out"=w234:errorcluster)  [unwired: 2 in, 4 out]
                  }
                  frame True {
                    # "Si SET Z manual"
                    n181 = local read "Settings Z"() -> (w245:T4)
                    n182 = Bundle By Name(cluster=w245, "targetField"="Target Z", "rampRate"="Rate Z") -> (w251:T4)
                    n183 = global write "cRIO_ZNB_AMI_GLOBALES.vi" "Target Z"("Target Z") -> ()
                    n184 = global write "cRIO_ZNB_AMI_GLOBALES.vi" "Rate Z"("Rate Z") -> ()
                    n185 = local write "Settings Z"(w251) -> ()
                    n186 = local read "ConfigZ"() -> (w249:T1)
                    n187 = global read "cRIO_ZNB_AMI_GLOBALES.vi" "EN"() -> (w246:bool)
                    n188 = call "AMI 430_Hardware_Module_Z AXIS.vi"("Enable"=w246, "Command"=AMI_430_Hardware_Module."SET  RAMPA", "error in (no error)"=w253, "Settings"=w251, "Comm Config In"=w249) -> ("error out"=w257:errorcluster)  [unwired: 2 in, 4 out]
                    n189 = call "Time Delay9"("error in (no error)"=w257, "Delay Time (s)"=w250) -> ("error out"=w256:errorcluster)  [unwired: 9 in]
                    n190 = call "AMI 430_Hardware_Module_Z AXIS.vi"("Enable"=w246, "Command"=AMI_430_Hardware_Module."SET CAMPO", "error in (no error)"=w256, "Settings"=w251, "Comm Config In"=w249) -> ("error out"=w252:errorcluster)  [unwired: 2 in, 4 out]
                    n191 = global write "cRIO_ZNB_AMI_GLOBALES.vi" "Remote SET Z"(FALSE ("Remote SET X")) -> ()
                    n192 = local write "SET Z"(FALSE ("Remote SET X")) -> ()
                  }
                }
                n193 = local write "Estado"("Cambio parámetros eje Z ..." ("String")) -> ()
              }
            }
          }
          frame "RAMP X" {
            n194 = global read "cRIO_ZNB_AMI_GLOBALES.vi" "Remote GO X"() -> (w262:bool)
            n195 = Or(x=w262, y="GO X") -> (x .or. y?=w261:bool)
            n196 = case shown="True" w261 {
              tunnel: w266 -> [w267 w272]
              tunnel: [w267 w271] -> w265
              tunnel: w263 -> [_ w270]
              tunnel: "GO X" -> [_ w269]
              frame False {
              }
              frame True {
                # "Si RAMP  X manual o remoto..."
                n197 = case shown="False" w269 {
                  tunnel: w272 -> [w277 w291]
                  tunnel: [w278 w290] -> w271
                  tunnel: w270 -> [w276 w289]
                  frame False {
                    # "Si RAMP X remoto"
                    n198 = global read "cRIO_ZNB_AMI_GLOBALES.vi" "rampingMode X"() -> (w282:u16)
                    n199 = local read "Settings X"() -> (w273:T4)
                    n200 = Bundle By Name(cluster=w273, "rampingMode"=w282) -> (w280:T4)
                    n201 = local write "Mode X"(w282) -> ()
                    n202 = local write "Settings X"(w280) -> ()
                    n203 = local read "ConfigX"() -> (w275:T1)
                    n204 = global read "cRIO_ZNB_AMI_GLOBALES.vi" "EN"() -> (w274:bool)
                    n205 = local write "GO X"(FALSE ("Remote SET X")) -> ()
                    n206 = global write "cRIO_ZNB_AMI_GLOBALES.vi" "Remote GO X"(FALSE ("Remote SET X")) -> ()
                    n207 = call "AMI 430_Hardware_Module_X AXIS.vi"("Enable"=w274, "Command"=AMI_430_Hardware_Module."SET RAMPING MODE", "error in (no error)"=w277, "Settings"=w280, "Comm Config In"=w275) -> ("error out"=w281:errorcluster)  [unwired: 2 in, 4 out]
                    n208 = call "Time Delay11"("error in (no error)"=w281, "Delay Time (s)"=w276) -> ("error out"=w278:errorcluster)  [unwired: 9 in]
                  }
                  frame True {
                    # "Si RAMP X manual"
                    n209 = local read "Settings X"() -> (w285:T4)
                    n210 = Bundle By Name(cluster=w285, "rampingMode"="Mode X") -> (w293:T4)
                    n211 = global write "cRIO_ZNB_AMI_GLOBALES.vi" "rampingMode X"("Mode X") -> ()
                    n212 = local write "Settings X"(w293) -> ()
                    n213 = local read "ConfigX"() -> (w287:T1)
                    n214 = global read "cRIO_ZNB_AMI_GLOBALES.vi" "EN"() -> (w286:bool)
                    n215 = local write "GO X"(FALSE ("Remote SET X")) -> ()
                    n216 = global write "cRIO_ZNB_AMI_GLOBALES.vi" "Remote GO X"(FALSE ("Remote SET X")) -> ()
                    n217 = call "AMI 430_Hardware_Module_X AXIS.vi"("Enable"=w286, "Command"=AMI_430_Hardware_Module."SET RAMPING MODE", "error in (no error)"=w291, "Settings"=w293, "Comm Config In"=w287) -> ("error out"=w294:errorcluster)  [unwired: 2 in, 4 out]
                    n218 = call "Time Delay6"("error in (no error)"=w294, "Delay Time (s)"=w289) -> ("error out"=w290:errorcluster)  [unwired: 9 in]
                  }
                }
                n219 = local write "Estado"("Cambio modo de rampa eje X ..." ("String")) -> ()
              }
            }
          }
          frame "RAMP Y" {
            n220 = global read "cRIO_ZNB_AMI_GLOBALES.vi" "Remote GO Y"() -> (w299:bool)
            n221 = Or(x=w299, y="GO Y") -> (x .or. y?=w298:bool)
            n222 = case shown="True" w298 {
              tunnel: w303 -> [w304 w309]
              tunnel: [w304 w308] -> w302
              tunnel: w300 -> [_ w307]
              tunnel: "GO Y" -> [_ w306]
              frame False {
              }
              frame True {
                # "Si RAMP  Y manual o remoto..."
                n223 = case shown="True" w306 {
                  tunnel: w309 -> [w314 w328]
                  tunnel: [w315 w327] -> w308
                  tunnel: w307 -> [w313 w326]
                  frame False {
                    # "Si RAMP Y remoto"
                    n224 = global read "cRIO_ZNB_AMI_GLOBALES.vi" "rampingMode Y"() -> (w319:u16)
                    n225 = local read "Settings Y"() -> (w310:T4)
                    n226 = Bundle By Name(cluster=w310, "rampingMode"=w319) -> (w317:T4)
                    n227 = local write "Mode Y"(w319) -> ()
                    n228 = local write "Settings Y"(w317) -> ()
                    n229 = local read "ConfigY"() -> (w312:T1)
                    n230 = global read "cRIO_ZNB_AMI_GLOBALES.vi" "EN"() -> (w311:bool)
                    n231 = global write "cRIO_ZNB_AMI_GLOBALES.vi" "Remote GO Y"(FALSE ("Remote SET X")) -> ()
                    n232 = local write "GO Y"(FALSE ("Remote SET X")) -> ()
                    n233 = call "AMI 430_Hardware_Module_Y AXIS.vi"("Enable"=w311, "Command"=AMI_430_Hardware_Module."SET RAMPING MODE", "error in (no error)"=w314, "Settings"=w317, "Comm Config In"=w312) -> ("error out"=w318:errorcluster)  [unwired: 2 in, 4 out]
                    n234 = call "Time Delay16"("error in (no error)"=w318, "Delay Time (s)"=w313) -> ("error out"=w315:errorcluster)  [unwired: 9 in]
                  }
                  frame True {
                    # "Si RAMP Y manual"
                    n235 = local read "Settings Y"() -> (w322:T4)
                    n236 = Bundle By Name(cluster=w322, "rampingMode"="Mode Y") -> (w330:T4)
                    n237 = global write "cRIO_ZNB_AMI_GLOBALES.vi" "rampingMode Y"("Mode Y") -> ()
                    n238 = local write "Settings Y"(w330) -> ()
                    n239 = local read "ConfigY"() -> (w324:T1)
                    n240 = global read "cRIO_ZNB_AMI_GLOBALES.vi" "EN"() -> (w323:bool)
                    n241 = global write "cRIO_ZNB_AMI_GLOBALES.vi" "Remote GO Y"(FALSE ("Remote SET X")) -> ()
                    n242 = local write "GO Y"(FALSE ("Remote SET X")) -> ()
                    n243 = call "AMI 430_Hardware_Module_Y AXIS.vi"("Enable"=w323, "Command"=AMI_430_Hardware_Module."SET RAMPING MODE", "error in (no error)"=w328, "Settings"=w330, "Comm Config In"=w324) -> ("error out"=w331:errorcluster)  [unwired: 2 in, 4 out]
                    n244 = call "Time Delay17"("error in (no error)"=w331, "Delay Time (s)"=w326) -> ("error out"=w327:errorcluster)  [unwired: 9 in]
                  }
                }
                n245 = local write "Estado"("Cambio modo de rampa eje Y ..." ("String")) -> ()
              }
            }
          }
          frame "RAMP Z" {
            n246 = global read "cRIO_ZNB_AMI_GLOBALES.vi" "Remote GO Z"() -> (w337:bool)
            n247 = Or(x=w337, y="GO Z") -> (x .or. y?=w336:bool)
            n248 = case shown="True" w336 {
              tunnel: w340 -> [w341 w346]
              tunnel: [w341 w345] -> w339
              tunnel: w338 -> [_ w344]
              tunnel: "GO Z" -> [_ w343]
              frame False {
              }
              frame True {
                # "Si RAMP  Z manual o remoto..."
                n249 = case shown="True" w343 {
                  tunnel: w346 -> [w351 w365]
                  tunnel: [w352 w364] -> w345
                  tunnel: w344 -> [w350 w363]
                  frame False {
                    # "Si RAMP X remoto"
                    n250 = global read "cRIO_ZNB_AMI_GLOBALES.vi" "rampingMode Z"() -> (w356:u16)
                    n251 = local read "Settings Z"() -> (w347:T4)
                    n252 = Bundle By Name(cluster=w347, "rampingMode"=w356) -> (w354:T4)
                    n253 = local write "Mode Z"(w356) -> ()
                    n254 = local write "Settings Z"(w354) -> ()
                    n255 = local read "ConfigZ"() -> (w349:T1)
                    n256 = global read "cRIO_ZNB_AMI_GLOBALES.vi" "EN"() -> (w348:bool)
                    n257 = global write "cRIO_ZNB_AMI_GLOBALES.vi" "Remote GO Z"(FALSE ("Remote SET X")) -> ()
                    n258 = local write "GO Z"(FALSE ("Remote SET X")) -> ()
                    n259 = call "AMI 430_Hardware_Module_Z AXIS.vi"("Enable"=w348, "Command"=AMI_430_Hardware_Module."SET RAMPING MODE", "error in (no error)"=w351, "Settings"=w354, "Comm Config In"=w349) -> ("error out"=w355:errorcluster)  [unwired: 2 in, 4 out]
                    n260 = call "Time Delay19"("error in (no error)"=w355, "Delay Time (s)"=w350) -> ("error out"=w352:errorcluster)  [unwired: 9 in]
                  }
                  frame True {
                    # "Si RAMP Z manual"
                    n261 = local read "Settings Z"() -> (w359:T4)
                    n262 = global write "cRIO_ZNB_AMI_GLOBALES.vi" "rampingMode Z"("Mode Z") -> ()
                    n263 = Bundle By Name(cluster=w359, "rampingMode"="Mode Z") -> (w367:T4)
                    n264 = local write "Settings Z"(w367) -> ()
                    n265 = local read "ConfigZ"() -> (w361:T1)
                    n266 = global read "cRIO_ZNB_AMI_GLOBALES.vi" "EN"() -> (w360:bool)
                    n267 = global write "cRIO_ZNB_AMI_GLOBALES.vi" "Remote GO Z"(FALSE ("Remote SET X")) -> ()
                    n268 = local write "GO Z"(FALSE ("Remote SET X")) -> ()
                    n269 = call "AMI 430_Hardware_Module_Z AXIS.vi"("Enable"=w360, "Command"=AMI_430_Hardware_Module."SET RAMPING MODE", "error in (no error)"=w365, "Settings"=w367, "Comm Config In"=w361) -> ("error out"=w368:errorcluster)  [unwired: 2 in, 4 out]
                    n270 = call "Time Delay20"("error in (no error)"=w368, "Delay Time (s)"=w363) -> ("error out"=w364:errorcluster)  [unwired: 9 in]
                  }
                }
                n271 = local write "Estado"("Cambio modo de rampa eje Z ..." ("String")) -> ()
              }
            }
          }
          frame "RAMP XYZ" {
            n272 = global read "cRIO_ZNB_AMI_GLOBALES.vi" "Remote GO XYZ"() -> (w373:bool)
            n273 = Or(x=w373, y="GO XYZ") -> (x .or. y?=w372:bool)
            n274 = case shown="True" w372 {
              tunnel: w377 -> [w378 w383]
              tunnel: [w378 w382] -> w376
              tunnel: w375 -> [_ w381]
              tunnel: "GO XYZ" -> [_ w380]
              frame False {
              }
              frame True {
                # "Si GO  XYZ manual o remoto..."
                n275 = case shown="True" w380 {
                  tunnel: w383 -> [w384 w388]
                  tunnel: [w384 w385] -> w382
                  tunnel: w381 -> [_ w389]
                  frame False {
                    # "Si RAMP XYZ remoto"
                  }
                  frame True {
                    # "Si GO  XYZ manual"
                    n276 = flat-sequence {
                      tunnel: w389 -> [w396]
                      tunnel: w388 -> [w390]
                      tunnel: [w396] -> w387
                      tunnel: [w390] -> w386
                      tunnel: w387 -> [w422]
                      tunnel: w386 -> [w434]
                      tunnel: [w411] -> w385
                      frame #0 {
                        w391 = u32 16716800 ("Color Box 2")
                        n277 = local read "cRate_X"() -> (w392:dbl)
                        n278 = local read "cTarget_X"() -> (w393:dbl)
                        n279 = local read "cRate_Y"() -> (w394:dbl)
                        n280 = local read "cTarget_Y"() -> (w395:dbl)
                        n281 = property on="Target X" class="DigNum (strict)"("NumText.TextColor"=w391) -> ()  [unwired: 2 in, 2 out]
                        n282 = property on="Rate X" class="DigNum (strict)"("NumText.TextColor"=w391) -> ()  [unwired: 2 in, 2 out]
                        n283 = property on="Target Y" class="DigNum (strict)"("NumText.TextColor"=w391) -> ()  [unwired: 2 in, 2 out]
                        n284 = property on="Rate Y" class="DigNum (strict)"("NumText.TextColor"=w391) -> ()  [unwired: 2 in, 2 out]
                        n285 = local write "Rate X"(w392) -> ()
                        n286 = local write "Target X"(w393) -> ()
                        n287 = local write "Rate Y"(w394) -> ()
                        n288 = local write "Target Y"(w395) -> ()
                      }
                      frame #1 {
                        w401 = AMI_430_Hardware_Module."SET RAMPING MODE" ("Command")
                        w400 = AMI_430_Hardware_Module."SET CAMPO" ("Command")
                        w399 = AMI_430_Hardware_Module."SET  RAMPA" ("Command")
                        n289 = local read "Target Y"() -> (w441:dbl)
                        n290 = local read "Target Z"() -> (w443:dbl)
                        n291 = local read "Rate Y"() -> (w440:dbl)
                        n292 = local read "Target X"() -> (w438:dbl)
                        n293 = local read "Rate Z"() -> (w444:dbl)
                        n294 = local read "Rate X"() -> (w437:dbl)
                        n295 = local read "Settings Y"() -> (w439:T4)
                        n296 = local read "Settings Z"() -> (w442:T4)
                        n297 = local read "Settings X"() -> (w435:T4)
                        n298 = Bundle By Name(cluster=w442, "targetField"=w443, "rampRate"=w444) -> (w419:T4)
                        n299 = global write "cRIO_ZNB_AMI_GLOBALES.vi" "Target Z"(w443) -> ()
                        n300 = global write "cRIO_ZNB_AMI_GLOBALES.vi" "Rate Z"(w444) -> ()
                        n301 = Bundle By Name(cluster=w439, "targetField"=w441, "rampRate"=w440) -> (w414:T4)
                        n302 = global write "cRIO_ZNB_AMI_GLOBALES.vi" "Target Y"(w441) -> ()
                        n303 = global write "cRIO_ZNB_AMI_GLOBALES.vi" "Rate Y"(w440) -> ()
                        n304 = Bundle By Name(cluster=w435, "targetField"=w438, "rampRate"=w437) -> (w412:T4)
                        n305 = global write "cRIO_ZNB_AMI_GLOBALES.vi" "Target X"(w438) -> ()
                        n306 = global write "cRIO_ZNB_AMI_GLOBALES.vi" "Rate X"(w437) -> ()
                        n307 = local write "Settings X"(w412) -> ()
                        n308 = local read "ConfigX"() -> (w404:T1)
                        n309 = local write "Settings Z"(w419) -> ()
                        n310 = local write "Settings Y"(w414) -> ()
                        n311 = local read "ConfigZ"() -> (w416:T1)
                        n312 = local read "ConfigY"() -> (w405:T1)
                        n313 = global read "cRIO_ZNB_AMI_GLOBALES.vi" "EN"() -> (w436:bool)
                        n314 = call "AMI 430_Hardware_Module_X AXIS.vi"("Enable"=w436, "Command"=w399, "error in (no error)"=w434, "Settings"=w412, "Comm Config In"=w404) -> ("error out"=w433:errorcluster)  [unwired: 2 in, 4 out]
                        n315 = global read "cRIO_ZNB_AMI_GLOBALES.vi" "EN"() -> (w431:bool)
                        n316 = call "AMI 430_Hardware_Module_Y AXIS.vi"("Enable"=w431, "Command"=w399, "error in (no error)"=w433, "Settings"=w414, "Comm Config In"=w405) -> ("error out"=w432:errorcluster)  [unwired: 2 in, 4 out]
                        n317 = global read "cRIO_ZNB_AMI_GLOBALES.vi" "EN"() -> (w430:bool)
                        n318 = call "AMI 430_Hardware_Module_Z AXIS.vi"("Enable"=w430, "Command"=w399, "error in (no error)"=w432, "Settings"=w419, "Comm Config In"=w416) -> ("error out"=w429:errorcluster)  [unwired: 2 in, 4 out]
                        n319 = call "Time Delay7"("error in (no error)"=w429, "Delay Time (s)"=w422) -> ("error out"=w421:errorcluster)  [unwired: 9 in]
                        n320 = global read "cRIO_ZNB_AMI_GLOBALES.vi" "EN"() -> (w426:bool)
                        n321 = call "AMI 430_Hardware_Module_X AXIS.vi"("Enable"=w426, "Command"=w400, "error in (no error)"=w421, "Settings"=w412, "Comm Config In"=w404) -> ("error out"=w425:errorcluster)  [unwired: 2 in, 4 out]
                        n322 = global read "cRIO_ZNB_AMI_GLOBALES.vi" "EN"() -> (w427:bool)
                        n323 = call "AMI 430_Hardware_Module_Y AXIS.vi"("Enable"=w427, "Command"=w400, "error in (no error)"=w425, "Settings"=w414, "Comm Config In"=w405) -> ("error out"=w424:errorcluster)  [unwired: 2 in, 4 out]
                        n324 = global read "cRIO_ZNB_AMI_GLOBALES.vi" "EN"() -> (w428:bool)
                        n325 = call "AMI 430_Hardware_Module_Z AXIS.vi"("Enable"=w428, "Command"=w400, "error in (no error)"=w424, "Settings"=w419, "Comm Config In"=w416) -> ("error out"=w423:errorcluster)  [unwired: 2 in, 4 out]
                        n326 = call "Time Delay10"("error in (no error)"=w423, "Delay Time (s)"=w422) -> ("error out"=w407:errorcluster)  [unwired: 9 in]
                        n327 = local read "Mode Z"() -> (w420:u16)
                        n328 = local read "Mode Y"() -> (w415:u16)
                        n329 = local read "Mode X"() -> (w413:u16)
                        n330 = Bundle By Name(cluster=w419, "rampingMode"=w420) -> (w418:T4)
                        n331 = global write "cRIO_ZNB_AMI_GLOBALES.vi" "rampingMode Z"(w420) -> ()
                        n332 = Bundle By Name(cluster=w414, "rampingMode"=w415) -> (w402:T4)
                        n333 = global write "cRIO_ZNB_AMI_GLOBALES.vi" "rampingMode Y"(w415) -> ()
                        n334 = Bundle By Name(cluster=w412, "rampingMode"=w413) -> (w403:T4)
                        n335 = global write "cRIO_ZNB_AMI_GLOBALES.vi" "rampingMode X"(w413) -> ()
                        n336 = local write "Settings Z"(w418) -> ()
                        n337 = local write "Settings Y"(w402) -> ()
                        n338 = local write "Settings X"(w403) -> ()
                        n339 = global read "cRIO_ZNB_AMI_GLOBALES.vi" "EN"() -> (w409:bool)
                        n340 = call "AMI 430_Hardware_Module_X AXIS.vi"("Enable"=w409, "Command"=w401, "error in (no error)"=w407, "Settings"=w403, "Comm Config In"=w404) -> ("error out"=w410:errorcluster)  [unwired: 2 in, 4 out]
                        n341 = global read "cRIO_ZNB_AMI_GLOBALES.vi" "EN"() -> (w408:bool)
                        n342 = call "AMI 430_Hardware_Module_Y AXIS.vi"("Enable"=w408, "Command"=w401, "error in (no error)"=w410, "Settings"=w402, "Comm Config In"=w405) -> ("error out"=w406:errorcluster)  [unwired: 2 in, 4 out]
                        n343 = global read "cRIO_ZNB_AMI_GLOBALES.vi" "EN"() -> (w417:bool)
                        n344 = call "AMI 430_Hardware_Module_Z AXIS.vi"("Enable"=w417, "Command"=w401, "error in (no error)"=w406, "Settings"=w418, "Comm Config In"=w416) -> ("error out"=w411:errorcluster)  [unwired: 2 in, 4 out]
                        n345 = global write "cRIO_ZNB_AMI_GLOBALES.vi" "Remote GO XYZ"(FALSE ("Remote SET X")) -> ()
                        n346 = local write "GO XYZ"(FALSE ("Remote SET X")) -> ()
                      }
                    }
                  }
                }
                n347 = local write "Estado"("Cambio parametros XYZ ..." ("String")) -> ()
              }
            }
          }
          frame "DESIMANAR X" {
            n348 = global read "cRIO_ZNB_AMI_GLOBALES.vi" "Remote DEMAG X"() -> (w447:bool)
            n349 = Or(x=w447, y="DEMAG X") -> (x .or. y?=w446:bool)
            n350 = case shown="True" w446 {
              tunnel: w451 -> [w452 w457]
              tunnel: [w452 w456] -> w450
              tunnel: w448 -> [_ w455]
              tunnel: "DEMAG X" -> [_ w454]
              frame False {
              }
              frame True {
                # "Si DEMAG  X manual o remoto..."
                n351 = case shown="True" w454 {
                  tunnel: w457 -> [w458 w472]
                  tunnel: [w458 w475] -> w456
                  tunnel: w455 -> [_ w463]
                  frame False {
                    # "Si RAMP X remoto"
                  }
                  frame True {
                    w474 = u16 0 items=["RAMP", "PAUSE", "MANUAL UP", "MANUAL DOWN", "ZERO"] ("rampingMode X 2")
                    # "Si RAMP X manual"
                    n352 = call "AMI_Desimana X axis.vi"("error in (no error)"=w472) -> ("error out"=w471:errorcluster, "resulting string X"=w473:string)  [unwired: 7 in]
                    n353 = call "AMI_Parse_Desimanar_X.vi"("error in (no error)"=w471, "String"=w473) -> ("error out"=w468:errorcluster, "X Wait secs"=w462:dbl, "X Rate"=w466:dbl, "X Steps"=w467:i32)  [unwired: 6 in]
                    n354 = local read "Settings X"() -> (w459:T4)
                    n355 = Bundle By Name(cluster=w459, "rampingMode"=w474) -> (w470:T4)
                    n356 = global write "cRIO_ZNB_AMI_GLOBALES.vi" "rampingMode X"(w474) -> ()
                    n357 = global read "cRIO_ZNB_AMI_GLOBALES.vi" "X field"() -> (w465:dbl)
                    n358 = local write "Mode X"(w474) -> ()
                    n359 = call "Demag_fields.vi"("error in (no error)"=w468, "Steps"=w467, "Field (T)"=w465) -> ("error out"=w469:errorcluster, "Fields"=w464:dbl[])  [unwired: 7 in]
                    n360 = local write "Settings X"(w470) -> ()
                    n361 = local read "ConfigX"() -> (w461:T1)
                    n362 = for {
                      tunnel: w463 -> [w483]
                      tunnel: w461 -> [w488]
                      tunnel: w470 -> [w487]
                      shift-right: [w481] -> w475
                      shift-left: w469 -> [w485]
                      tunnel: w466 -> [w478]
                      tunnel: w464 -> [w477] mode=indexing
                      tunnel: w462 -> [w480]
                      tunnel: [FALSE ("Remote SET X")] -> w460
                      n363 = Bundle By Name(cluster=w487, "targetField"=w477, "rampRate"=w478) -> (w486:T4)
                      n364 = global write "cRIO_ZNB_AMI_GLOBALES.vi" "Target X"(w477) -> ()
                      n365 = local write "Target X"(w477) -> ()
                      n366 = global write "cRIO_ZNB_AMI_GLOBALES.vi" "Rate X"(w478) -> ()
                      n367 = local write "Rate X"(w478) -> ()
                      n368 = local write "Settings X"(w486) -> ()
                      n369 = global read "cRIO_ZNB_AMI_GLOBALES.vi" "EN"() -> (w476:bool)
                      n370 = call "AMI 430_Hardware_Module_X AXIS.vi"("Enable"=w476, "Command"=AMI_430_Hardware_Module."SET  RAMPA", "error in (no error)"=w485, "Settings"=w486, "Comm Config In"=w488) -> ("error out"=w493:errorcluster)  [unwired: 2 in, 4 out]
                      n371 = call "Time Delay31"("error in (no error)"=w493, "Delay Time (s)"=w483) -> ("error out"=w494:errorcluster)  [unwired: 9 in]
                      n372 = call "AMI 430_Hardware_Module_X AXIS.vi"("Enable"=w476, "Command"=AMI_430_Hardware_Module."SET CAMPO", "error in (no error)"=w494, "Settings"=w486, "Comm Config In"=w488) -> ("error out"=w490:errorcluster)  [unwired: 2 in, 4 out]
                      n373 = call "Time Delay32"("error in (no error)"=w490, "Delay Time (s)"=w483) -> ("error out"=w489:errorcluster)  [unwired: 9 in]
                      n374 = call "AMI 430_Hardware_Module_X AXIS.vi"("Enable"=w476, "Command"=AMI_430_Hardware_Module."SET RAMPING MODE", "error in (no error)"=w489, "Settings"=w486, "Comm Config In"=w488) -> ("error out"=w496:errorcluster)  [unwired: 2 in, 4 out]
                      n375 = call "Time Delay25"("error in (no error)"=w496, "Delay Time (s)"=w483) -> ("error out"=w484:errorcluster)  [unwired: 9 in]
                      n376 = while {
                        shift-right: [w502] -> w482
                        shift-left: w484 -> [w504]
                        tunnel: w483 -> [w501]
                        stop <- w499 stop-if-true
                        w507 = T3 1 items=["Unknown", "RAMPING to target field/current", "HOLDING at the target field/current", "PAUSED", "Ramping in MANUAL UP mode", "Ramping in MANUAL DOWN mode", "ZEROING CURRENT (in progress)", "Quench detected", "At ZERO current", "Heating persistent switch", "Cooling persistent switch", "External Rampdown active"] ("y")
                        n377 = global read "cRIO_ZNB_AMI_GLOBALES.vi" "EN"() -> (w497:bool)
                        n378 = property on="Refresh" class="Bool (strict)"(error in=w504, "Value"=TRUE ("Refresh")) -> (error out=w509:errorcluster)  [unwired: 1 in, 1 out]
                        n379 = call "AMI 430_Hardware_Module_X AXIS.vi"("Enable"=w497, "Command"=AMI_430_Hardware_Module."READ CAMPO", "error in (no error)"=w509) -> ("error out"=w514:errorcluster, "magneticField"=w517:dbl)  [unwired: 4 in, 3 out]
                        n380 = call "AMI 430_Hardware_Module_X AXIS.vi"("Enable"=w497, "Command"=AMI_430_Hardware_Module."STATUS", "error in (no error)"=w514) -> ("error out"=w508:errorcluster, "state"=w506:T3)  [unwired: 4 in, 3 out]
                        n381 = global write "cRIO_ZNB_AMI_GLOBALES.vi" "X state"(w506) -> ()
                        n382 = local write "X state"(w506) -> ()
                        n383 = property on="Refresh" class="Bool (strict)"(error in=w508, "Value"=FALSE ("Refresh")) -> (error out=w503:errorcluster)  [unwired: 1 in, 1 out]
                        n384 = global read "cRIO_ZNB_AMI_GLOBALES.vi" "Z field"() -> (w515:dbl)
                        n385 = global read "cRIO_ZNB_AMI_GLOBALES.vi" "Y field"() -> (w516:dbl)
                        n386 = global write "cRIO_ZNB_AMI_GLOBALES.vi" "X field"(w517) -> ()
                        n387 = local write "X field"(w517) -> ()
                        n388 = Equal?(x=w506, y=w507) -> (x = y?=w505:bool)
                        n389 = Bundle("Z field"=w515, "Y field"=w516, "magneticField"=w517) -> (w518:T7)  [unwired: 1 in]
                        n390 = local write "X ramping"(w505) -> ()
                        n391 = global write "cRIO_ZNB_AMI_GLOBALES.vi" "X ramping"(w505) -> ()
                        n392 = local write "Waveform Chart"(w518) -> ()
                        n393 = call "Time Delay33"("error in (no error)"=w503, "Delay Time (s)"=w501) -> ("error out"=w502:errorcluster)  [unwired: 9 in]
                        n394 = Not(x=w505) -> (.not. x?=w500:bool)
                        n395 = Or(x=w500, y=FALSE ("Refresh")) -> (x .or. y?=w499:bool)
                      }
                      n396 = call "Time Delay34"("error in (no error)"=w482, "Delay Time (s)"=w480) -> ("error out"=w481:errorcluster)  [unwired: 9 in]
                    }
                    n397 = global write "cRIO_ZNB_AMI_GLOBALES.vi" "Remote DEMAG X"(w460) -> ()
                    n398 = local write "DEMAG X"(w460) -> ()
                  }
                }
                n399 = local write "Estado"("Desmagnetizando eje X ... ESPERE..." ("String")) -> ()
              }
            }
          }
          frame "DESIMANAR Y" {
            n400 = global read "cRIO_ZNB_AMI_GLOBALES.vi" "Remote DEMAG Y"() -> (w521:bool)
            n401 = Or(x=w521, y="DEMAG Y") -> (x .or. y?=w520:bool)
            n402 = case shown="True" w520 {
              tunnel: w525 -> [w526 w531]
              tunnel: [w526 w530] -> w524
              tunnel: w522 -> [_ w529]
              tunnel: "DEMAG Y" -> [_ w528]
              frame False {
              }
              frame True {
                # "Si DEMAG  Y manual o remoto..."
                n403 = case shown="True" w528 {
                  tunnel: w531 -> [w532 w546]
                  tunnel: [w532 w549] -> w530
                  tunnel: w529 -> [_ w537]
                  frame False {
                    # "Si RAMP Y remoto"
                  }
                  frame True {
                    w548 = u16 0 items=["RAMP", "PAUSE", "MANUAL UP", "MANUAL DOWN", "ZERO"] ("rampingMode X 2")
                    # "Si RAMP Y manual"
                    n404 = call "AMI_Desimana Y axis.vi"("error in (no error)"=w546) -> ("error out"=w545:errorcluster, "resulting string Y"=w547:string)  [unwired: 7 in]
                    n405 = call "AMI_Parse_Desimanar_Y.vi"("error in (no error)"=w545, "String"=w547) -> ("error out"=w542:errorcluster, "Y Wait secs"=w536:i32, "Y Rate"=w540:dbl, "Y Steps"=w541:i32)  [unwired: 6 in]
                    n406 = local read "Settings Y"() -> (w533:T4)
                    n407 = Bundle By Name(cluster=w533, "rampingMode"=w548) -> (w544:T4)
                    n408 = global write "cRIO_ZNB_AMI_GLOBALES.vi" "rampingMode Y"(w548) -> ()
                    n409 = global read "cRIO_ZNB_AMI_GLOBALES.vi" "Y field"() -> (w539:dbl)
                    n410 = local write "Mode Y"(w548) -> ()
                    n411 = call "Demag_fields.vi"("error in (no error)"=w542, "Steps"=w541, "Field (T)"=w539) -> ("error out"=w543:errorcluster, "Fields"=w538:dbl[])  [unwired: 7 in]
                    n412 = local write "Settings Y"(w544) -> ()
                    n413 = local read "ConfigY"() -> (w535:T1)
                    n414 = for {
                      tunnel: w537 -> [w557]
                      tunnel: w535 -> [w562]
                      tunnel: w544 -> [w561]
                      shift-right: [w555] -> w549
                      shift-left: w543 -> [w559]
                      tunnel: w540 -> [w552]
                      tunnel: w538 -> [w551] mode=indexing
                      tunnel: w536 -> [w554]
                      tunnel: [FALSE ("Remote SET X")] -> w534
                      n415 = Bundle By Name(cluster=w561, "targetField"=w551, "rampRate"=w552) -> (w560:T4)
                      n416 = global write "cRIO_ZNB_AMI_GLOBALES.vi" "Target Y"(w551) -> ()
                      n417 = local write "Target Y"(w551) -> ()
                      n418 = global write "cRIO_ZNB_AMI_GLOBALES.vi" "Rate Y"(w552) -> ()
                      n419 = local write "Rate Y"(w552) -> ()
                      n420 = local write "Settings Y"(w560) -> ()
                      n421 = global read "cRIO_ZNB_AMI_GLOBALES.vi" "EN"() -> (w550:bool)
                      n422 = call "AMI 430_Hardware_Module_Y AXIS.vi"("Enable"=w550, "Command"=AMI_430_Hardware_Module."SET  RAMPA", "error in (no error)"=w559, "Settings"=w560, "Comm Config In"=w562) -> ("error out"=w567:errorcluster)  [unwired: 2 in, 4 out]
                      n423 = call "Time Delay21"("error in (no error)"=w567, "Delay Time (s)"=w557) -> ("error out"=w568:errorcluster)  [unwired: 9 in]
                      n424 = call "AMI 430_Hardware_Module_Y AXIS.vi"("Enable"=w550, "Command"=AMI_430_Hardware_Module."SET CAMPO", "error in (no error)"=w568, "Settings"=w560, "Comm Config In"=w562) -> ("error out"=w564:errorcluster)  [unwired: 2 in, 4 out]
                      n425 = call "Time Delay22"("error in (no error)"=w564, "Delay Time (s)"=w557) -> ("error out"=w563:errorcluster)  [unwired: 9 in]
                      n426 = call "AMI 430_Hardware_Module_Y AXIS.vi"("Enable"=w550, "Command"=AMI_430_Hardware_Module."SET RAMPING MODE", "error in (no error)"=w563, "Settings"=w560, "Comm Config In"=w562) -> ("error out"=w570:errorcluster)  [unwired: 2 in, 4 out]
                      n427 = call "Time Delay18"("error in (no error)"=w570, "Delay Time (s)"=w557) -> ("error out"=w558:errorcluster)  [unwired: 9 in]
                      n428 = while {
                        shift-right: [w578] -> w556
                        shift-left: w558 -> [w580]
                        tunnel: w557 -> [w577]
                        stop <- w575 stop-if-true
                        w583 = T3 1 items=["Unknown", "RAMPING to target field/current", "HOLDING at the target field/current", "PAUSED", "Ramping in MANUAL UP mode", "Ramping in MANUAL DOWN mode", "ZEROING CURRENT (in progress)", "Quench detected", "At ZERO current", "Heating persistent switch", "Cooling persistent switch", "External Rampdown active"] ("y")
                        n429 = global read "cRIO_ZNB_AMI_GLOBALES.vi" "EN"() -> (w571:bool)
                        n430 = property on="Refresh" class="Bool (strict)"(error in=w580, "Value"=TRUE ("Refresh")) -> (error out=w585:errorcluster)  [unwired: 1 in, 1 out]
                        n431 = call "AMI 430_Hardware_Module_Y AXIS.vi"("Enable"=w571, "Command"=AMI_430_Hardware_Module."READ CAMPO", "error in (no error)"=w585) -> ("error out"=w590:errorcluster, "magneticField"=w572:dbl)  [unwired: 4 in, 3 out]
                        n432 = call "AMI 430_Hardware_Module_Y AXIS.vi"("Enable"=w571, "Command"=AMI_430_Hardware_Module."STATUS", "error in (no error)"=w590) -> ("error out"=w584:errorcluster, "state"=w582:T3)  [unwired: 4 in, 3 out]
                        n433 = global write "cRIO_ZNB_AMI_GLOBALES.vi" "Y state"(w582) -> ()
                        n434 = local write "Y state"(w582) -> ()
                        n435 = property on="Refresh" class="Bool (strict)"(error in=w584, "Value"=FALSE ("Refresh")) -> (error out=w579:errorcluster)  [unwired: 1 in, 1 out]
                        n436 = global read "cRIO_ZNB_AMI_GLOBALES.vi" "Z field"() -> (w591:dbl)
                        n437 = global write "cRIO_ZNB_AMI_GLOBALES.vi" "Y field"(w572) -> ()
                        n438 = global read "cRIO_ZNB_AMI_GLOBALES.vi" "X field"() -> (w573:dbl)
                        n439 = local write "Y field"(w572) -> ()
                        n440 = Equal?(x=w582, y=w583) -> (x = y?=w581:bool)
                        n441 = Bundle("Z field"=w591, "magneticField"=w572, "X field"=w573) -> (w592:T8)  [unwired: 1 in]
                        n442 = local write "Y ramping"(w581) -> ()
                        n443 = global write "cRIO_ZNB_AMI_GLOBALES.vi" "Y ramping"(w581) -> ()
                        n444 = local write "Waveform Chart"(w592) -> ()
                        n445 = call "Time Delay23"("error in (no error)"=w579, "Delay Time (s)"=w577) -> ("error out"=w578:errorcluster)  [unwired: 9 in]
                        n446 = Not(x=w581) -> (.not. x?=w576:bool)
                        n447 = Or(x=w576, y=FALSE ("Refresh")) -> (x .or. y?=w575:bool)
                      }
                      n448 = call "Time Delay24"("error in (no error)"=w556, "Delay Time (s)"=w554) -> ("error out"=w555:errorcluster)  [unwired: 9 in]
                    }
                    n449 = local write "DEMAG Y"(w534) -> ()
                    n450 = global write "cRIO_ZNB_AMI_GLOBALES.vi" "Remote DEMAG Y"(w534) -> ()
                  }
                }
                n451 = local write "Estado"("Desmagnetizando eje Y ... ESPERE..." ("String")) -> ()
              }
            }
          }
          frame "DESIMANAR Z" {
            n452 = global read "cRIO_ZNB_AMI_GLOBALES.vi" "Remote DEMAG Z"() -> (w595:bool)
            n453 = Or(x=w595, y="DEMAG Z") -> (x .or. y?=w594:bool)
            n454 = case shown="True" w594 {
              tunnel: w599 -> [w600 w605]
              tunnel: [w600 w604] -> w598
              tunnel: w596 -> [_ w603]
              tunnel: "DEMAG Z" -> [_ w602]
              frame False {
              }
              frame True {
                # "Si DEMAG  Z manual o remoto..."
                n455 = case shown="True" w602 {
                  tunnel: w605 -> [w606 w620]
                  tunnel: [w606 w623] -> w604
                  tunnel: w603 -> [_ w611]
                  frame False {
                    # "Si RAMP Z remoto"
                  }
                  frame True {
                    w622 = u16 0 items=["RAMP", "PAUSE", "MANUAL UP", "MANUAL DOWN", "ZERO"] ("rampingMode X 2")
                    # "Si RAMP Z manual"
                    n456 = call "AMI_Desimana Z axis.vi"("error in (no error)"=w620) -> ("error out"=w619:errorcluster, "resulting string Z"=w621:string)  [unwired: 7 in]
                    n457 = call "AMI_Parse_Desimanar_Z.vi"("error in (no error)"=w619, "String"=w621) -> ("error out"=w616:errorcluster, "Z Wait secs"=w610:i32, "Z Rate"=w614:dbl, "Z Steps"=w615:i32)  [unwired: 6 in]
                    n458 = local read "Settings Z"() -> (w607:T4)
                    n459 = Bundle By Name(cluster=w607, "rampingMode"=w622) -> (w618:T4)
                    n460 = global write "cRIO_ZNB_AMI_GLOBALES.vi" "rampingMode Z"(w622) -> ()
                    n461 = global read "cRIO_ZNB_AMI_GLOBALES.vi" "Z field"() -> (w613:dbl)
                    n462 = local write "Mode Z"(w622) -> ()
                    n463 = call "Demag_fields.vi"("error in (no error)"=w616, "Steps"=w615, "Field (T)"=w613) -> ("error out"=w617:errorcluster, "Fields"=w612:dbl[])  [unwired: 7 in]
                    n464 = local write "Settings Z"(w618) -> ()
                    n465 = local read "ConfigZ"() -> (w609:T1)
                    n466 = for {
                      tunnel: w611 -> [w631]
                      tunnel: w609 -> [w636]
                      tunnel: w618 -> [w635]
                      shift-right: [w629] -> w623
                      shift-left: w617 -> [w633]
                      tunnel: w614 -> [w626]
                      tunnel: w612 -> [w625] mode=indexing
                      tunnel: w610 -> [w628]
                      tunnel: [FALSE ("Remote SET X")] -> w608
                      n467 = Bundle By Name(cluster=w635, "targetField"=w625, "rampRate"=w626) -> (w634:T4)
                      n468 = global write "cRIO_ZNB_AMI_GLOBALES.vi" "Target Z"(w625) -> ()
                      n469 = local write "Target Z"(w625) -> ()
                      n470 = global write "cRIO_ZNB_AMI_GLOBALES.vi" "Rate Z"(w626) -> ()
                      n471 = local write "Rate Z"(w626) -> ()
                      n472 = local write "Settings Z"(w634) -> ()
                      n473 = global read "cRIO_ZNB_AMI_GLOBALES.vi" "EN"() -> (w624:bool)
                      n474 = call "AMI 430_Hardware_Module_Z AXIS.vi"("Enable"=w624, "Command"=AMI_430_Hardware_Module."SET  RAMPA", "error in (no error)"=w633, "Settings"=w634, "Comm Config In"=w636) -> ("error out"=w641:errorcluster)  [unwired: 2 in, 4 out]
                      n475 = call "Time Delay27"("error in (no error)"=w641, "Delay Time (s)"=w631) -> ("error out"=w642:errorcluster)  [unwired: 9 in]
                      n476 = call "AMI 430_Hardware_Module_Z AXIS.vi"("Enable"=w624, "Command"=AMI_430_Hardware_Module."SET CAMPO", "error in (no error)"=w642, "Settings"=w634, "Comm Config In"=w636) -> ("error out"=w638:errorcluster)  [unwired: 2 in, 4 out]
                      n477 = call "Time Delay28"("error in (no error)"=w638, "Delay Time (s)"=w631) -> ("error out"=w637:errorcluster)  [unwired: 9 in]
                      n478 = call "AMI 430_Hardware_Module_Z AXIS.vi"("Enable"=w624, "Command"=AMI_430_Hardware_Module."SET RAMPING MODE", "error in (no error)"=w637, "Settings"=w634, "Comm Config In"=w636) -> ("error out"=w644:errorcluster)  [unwired: 2 in, 4 out]
                      n479 = call "Time Delay26"("error in (no error)"=w644, "Delay Time (s)"=w631) -> ("error out"=w632:errorcluster)  [unwired: 9 in]
                      n480 = while {
                        shift-right: [w652] -> w630
                        shift-left: w632 -> [w654]
                        tunnel: w631 -> [w651]
                        stop <- w649 stop-if-true
                        w657 = T3 1 items=["Unknown", "RAMPING to target field/current", "HOLDING at the target field/current", "PAUSED", "Ramping in MANUAL UP mode", "Ramping in MANUAL DOWN mode", "ZEROING CURRENT (in progress)", "Quench detected", "At ZERO current", "Heating persistent switch", "Cooling persistent switch", "External Rampdown active"] ("y")
                        n481 = global read "cRIO_ZNB_AMI_GLOBALES.vi" "EN"() -> (w645:bool)
                        n482 = property on="Refresh" class="Bool (strict)"(error in=w654, "Value"=TRUE ("Refresh")) -> (error out=w659:errorcluster)  [unwired: 1 in, 1 out]
                        n483 = call "AMI 430_Hardware_Module_Z AXIS.vi"("Enable"=w645, "Command"=AMI_430_Hardware_Module."READ CAMPO", "error in (no error)"=w659) -> ("error out"=w664:errorcluster, "magneticField"=w647:dbl)  [unwired: 4 in, 3 out]
                        n484 = call "AMI 430_Hardware_Module_Z AXIS.vi"("Enable"=w645, "Command"=AMI_430_Hardware_Module."STATUS", "error in (no error)"=w664) -> ("error out"=w658:errorcluster, "state"=w656:T3)  [unwired: 4 in, 3 out]
                        n485 = global write "cRIO_ZNB_AMI_GLOBALES.vi" "Z state"(w656) -> ()
                        n486 = local write "Z state"(w656) -> ()
                        n487 = property on="Refresh" class="Bool (strict)"(error in=w658, "Value"=FALSE ("Refresh")) -> (error out=w653:errorcluster)  [unwired: 1 in, 1 out]
                        n488 = global write "cRIO_ZNB_AMI_GLOBALES.vi" "Z field"(w647) -> ()
                        n489 = global read "cRIO_ZNB_AMI_GLOBALES.vi" "Y field"() -> (w665:dbl)
                        n490 = global read "cRIO_ZNB_AMI_GLOBALES.vi" "X field"() -> (w646:dbl)
                        n491 = local write "Z field"(w647) -> ()
                        n492 = Equal?(x=w656, y=w657) -> (x = y?=w655:bool)
                        n493 = Bundle("magneticField"=w647, "Y field"=w665, "X field"=w646) -> (w666:T9)  [unwired: 1 in]
                        n494 = local write "Z ramping"(w655) -> ()
                        n495 = global write "cRIO_ZNB_AMI_GLOBALES.vi" "Z ramping"(w655) -> ()
                        n496 = local write "Waveform Chart"(w666) -> ()
                        n497 = call "Time Delay29"("error in (no error)"=w653, "Delay Time (s)"=w651) -> ("error out"=w652:errorcluster)  [unwired: 9 in]
                        n498 = Not(x=w655) -> (.not. x?=w650:bool)
                        n499 = Or(x=w650, y=FALSE ("Refresh")) -> (x .or. y?=w649:bool)
                      }
                      n500 = call "Time Delay30"("error in (no error)"=w630, "Delay Time (s)"=w628) -> ("error out"=w629:errorcluster)  [unwired: 9 in]
                    }
                    n501 = local write "DEMAG Z"(w608) -> ()
                    n502 = global write "cRIO_ZNB_AMI_GLOBALES.vi" "Remote DEMAG Z"(w608) -> ()
                  }
                }
                n503 = local write "Estado"("Desmagnetizando eje Z ... ESPERE..." ("String")) -> ()
              }
            }
          }
        }
        "Command" <- w62
        n504 = global read "cRIO_ZNB_AMI_GLOBALES.vi" "stopMagneticField"() -> (w69:bool)
        n505 = Unbundle By Name(w64) -> ("status"=→"Error":bool)
        n506 = call <vilib>:"Clear Errors.vi"("error in (no error)"=w64) -> ("error out"=w67:errorcluster)  [unwired: 5 in, 1 out]
        n507 = control-ref of="This VI"() -> (w70:refnum<vi>)
        n508 = Or(x="stop", y=w69) -> (x .or. y?=w72:bool)
        "Ciclo" <- w66
      }
      "Error Out" <- w58
      n509 = global write "cRIO_ZNB_AMI_GLOBALES.vi" "stopMagneticField"(w59) -> ()
      n510 = invoke class="VI" method="FP.Close"(reference=w60) -> ()  [unwired: 2 in, 3 out]
      "cRate_Y" <- 0.1 ("eRate_Y")
      "cTarget_Y" <- 0.0 ("eTarget_Y")
      "cRate_X" <- 0.1 ("eRate_X")
      "cTarget_X" <- 0.0 ("eTarget_X")
    }
  }
  n511 = global write "cRIO_ZNB_AMI_GLOBALES.vi" "x"(0.0 ("x")) -> ()
  n512 = global write "cRIO_ZNB_AMI_GLOBALES.vi" "y"(0.0 ("y")) -> ()
  "Estado" <- w3
